vi "VMI_Main_Events.vi"() -> ()   [LabVIEW 2018]
uses:
  <vilib>/vision/Image Controls.llb/IMAQ Image.ctl
  Type defs/TRPES_save_cluster.ctl
  <vilib>/userdefined/High Color/IMAQdx.ctl
  Type defs/Ref_cluster.ctl
  Type defs/Image_info.ctl
  Type defs/PI_delay_settings_alt.ctl
  Type defs/FileAcq_v1_Ctrl.ctl
  Type defs/Scan_ctrl.ctl
  Type defs/VMI_camera_contrl.ctl
  Type defs/DAQ_set_Ctrl.ctl
  Type defs/DAQ_Shutter_Ctrl.ctl
  Type defs/DAQ_AI_Ctrl.ctl
  Type defs/VMI_peak_out.ctl
  Type defs/IO_settings_ctrl.ctl
  Type defs/Header_infor_IF32.ctl
  <vilib>/DAQmx/write.llb/DAQmx Write (Digital 1D Bool NChan 1Samp 1Line).vi
  <vilib>/DAQmx/miscellaneous.llb/DAQmx Fill In Error Info.vi
panel:
  out "Peaks":T1[](array[typedef])
  out "Stage Position":dbl=50.0
  out "Delay Moving":bool
  in  "Files to Save":bool[](array[boolean])
  in  "Shutter2":bool
  in  "Shutter1":bool
  in  "Stop All":bool
  in  "Savechoose":bool caption="Choose save name?"
  out "Autosave?":bool
  in  "Save All":bool
  out "Running":bool
  out "Setup?":bool
  in  "Stop Collect":bool
  in  "New Collect":bool
  in  "Butt_Set":bool
  out "Information":string
  out "Hist_full":dbl[][][](array[numeric])
  in  "Collect":bool
  out "Peak Array":cluster{"X":sgl, "Y":sgl}[][](array[cluster])
  out "size(s) 3":i32
  out "size(s) 2":i32
  out "size(s)":i32
  out "Background 2":cluster{"X":sgl, "Y":sgl}[](array[cluster])
  out "Signal Background":cluster{"X":sgl, "Y":sgl}[](array[cluster])
  out "Background 1":cluster{"X":sgl, "Y":sgl}[](array[cluster])
  out "AI err":dbl[][](array[numeric])
  out "AI in":dbl[][](array[numeric])
  out "Big_image Array":i16[][][](array[numeric])
  out "Histogram_array":i32[][](array[numeric])
  in  "Bakc Image2":i16[][](array[numeric])
  in  "Bakc Image":i16[][](array[numeric])
  in  "Signal Image":i16[][](array[numeric])
  in  "Ref Cluster 1":T2
  out "Session Out":T3
  out "Queue Check":bool
  out "Queue Array":T4[](array[typedef])
  out "Image types Bool":bool[](array[boolean])
  out "Image Set":T5
  out "Points per image":i32[](array[numeric])
  in  "Error In":errorcluster
  out "Error Out":errorcluster
  in  "Tab Control":T6(tab)
  out "Count Rate / s":dbl
  in  "Delay Display":u16(ring) items=["Signal", "Background 1", "Background 2"]
  out "Delay":u8(slide) scale=0.0..4.0
  out "Current Image 3":T5(plugin-control)
  in  "Centroiding":u16(ring) items=["None", "x2"]
  in  "Image Options":u16(ring) items=["Last image", "Real Time", "Summed Image", "Background", "Background 2"]
  in  "Camera Rate / Hz":i32=50
  out "Collection Results":T7
  out "Counts per image":cluster{"X":dbl[], "Y":dbl[]}[](graph)
  in  "Acquire Time":i32=1 caption="How long to Acquire Image / s"
  in  "Total Acquires":i32=10000 caption="How many complete Acquires"
  out "max value":i16
  out "Delay Loop":i32
  out "Total Loop":i32
  in  "Save_Files":cluster{"Files to Save":bool[]}={"Files to Save"=[TRUE, TRUE, TRUE, TRUE]}
  in  "Image Info Acqu":T8={"X size"=782.0, "Y size"=582.0, "Centroiding"=1.0}
  in  "Database":bool
  in  "Log File":bool=TRUE
  in  "Slack":bool
  in  "Delay List":string[][](table)
  out "Delay Scan Steps":i32
  in  "Scan Set up":T9={"Scan Type"=0, "Collection Information File Path"=path "", "Chemical"="Xenon", "Comments"="", "Collection Time / s"=60, "Number Acquires"=1, "How long to acquire"=100} {"Scan Type" items=["Normal Collection - 1 Colour", "Normal Collection - 2 Colour", "Delay Scan - 2 colour", "Accurate Delay Scan - 2 Colour", "Settings file"]}
  in  "Collection Information":T10[](array[typedef])=[{"Type"="Signal and Background", "LaserWave1"=0.0, "Shutter1"=TRUE, "LaserWave2"=0.0, "Shutter2"=FALSE, "FileEnd"="_SignalBack", "Collect"=TRUE}]
  in  "Delay Cluster":T11={"System no."=0, "Identification"="", "Device ID out"=0, "Postion / mm"=[], "SN out"="", "Movement Range"=[], "Conn. Axes"=[], "Target Position / mm"=50.0, "Velocity / mm s^-1"=0.15, "Set-up"=FALSE, "Moving"=FALSE, "Step Size / mm "=0.15, "Stage Number"=0, "Polling Time /ms"=0, "Delay Scan?"=FALSE, "Accurate Scan"=FALSE, "CmdMovDelay"=FALSE, "CmdStopDelay"=FALSE, "Delay List"=[["Number", "Target / mm", "Relative Integration Time"]], "Scan Start /mm"=50.0, "Scan End / mm"=80.0}
  in  "Save Options":T12={"Auto Save"=FALSE, "Main Directory"=path "C:/Data", "Current File Date and endings"="", "Save Path"=path "C:/Data", "Backup Path"=path "Z:/Research_Projects/Photochemistry", "Extra Dir Information"="", "Remote"=TRUE}
  out "Last Slack":string
  in  "Loops per Save":i32
  in  "DAQ Settings":T13={"Shutters Settings"=[{"Name"="Shutter 1", "DAQ Channel/line"="Dev1/port0/line0", "Active"=TRUE}, {"Name"="Shutter 2", "DAQ Channel/line"="Dev1/port0/line1", "Active"=TRUE}], "Shutter Task"="Shutters_spare", "Acquire Settings"=[{"Name"="Power", "DAQ Channel/line"="Dev1/ai0", "Max V"=5.0, "Min V"=-5.0, "input terminal configuration"=10106, "Active"=TRUE}, {"Name"="Pressure 1", "DAQ Channel/line"="Dev1/ai1", "Max V"=5.0, "Min V"=-5.0, "input terminal configuration"=10106, "Active"=TRUE}, {"Name"="Pressure 2", "DAQ Channel/line"="Dev1/ai2", "Max V"=5.0, "Min V"=-5.0, "input terminal configuration"=10106, "Active"=TRUE}], "AI Task"="Acquire", "Sample mode"=10123, "Number of Samples"=100, "Rate"=1000.0, "AI Name"="Acquire", "DO Name"="Shutters"} {"Sample mode" items=["Finite Samples"=10178, "Continuous Samples"=10123, "Hardware Timed Single Point"=12522]; "Acquire Settings"."input terminal configuration" items=["default"=-1, "RSE"=10083, "NRSE"=10078, "Differential"=10106, "Pseudodifferential"=12529]}
  in  "Camera Settings":T16={"Run Options"=0, "Run Mode"=0, "Attributes"="[NIIMAQ_HEADER]\nType = 2\nVersion = 8\n\n[CAMERA_DATA]\nAcquisitionAttributes::VideoMode = \"Format 7, Mode 0, 782 x 582\"\nAcquisitionAttributes::OffsetX = \"0\"\nAcquisitionAttributes::OffsetY = \"0\"\nAcquisitionAttributes::Width = \"782\"\nAcquisitionAttributes::Height = \"582\"\nAcquisitionAttributes::Bayer::Algorithm = \"Bilinear\"\nAcquisitionAttributes::Bayer::GainB = \"1\"\nAcquisitionAttributes::Bayer::GainG = \"1\"\nAcquisitionAttributes::Bayer::GainR = \"1\"\nAcquisitionAttributes::Bayer::Pattern = \"Use hardware value\"\nAcquisitionAttributes::BitsPerPixel = \"Use hardware value\"\nAcquisitionAttributes::Controller::DesiredStreamChannel = \"0\"\nAcquisitionAttributes::Controller::StreamChannelMode = \"Automatic\"\nAcquisitionAttributes::IgnoreFirstFrame = \"false\"\nAcquisitionAttributes::ImageDecoderCopyMode = \"Auto\"\nAcquisitionAttributes::OutputImageType = \"Auto\"\nAcquisitionAttributes::OverwriteMode = \"Get Newest\"\nAcquisitionAttributes::PixelSignedness = \"Signed\"\nAcquisitionAttributes::ReceiveTimestampMode = \"None\"\nAcquisitionAttributes::ReserveDualPackets = \"false\"\nAcquisitionAttributes::ShiftPixelBits = \"false\"\nAcquisitionAttributes::Speed = \"400 Mbps\"\nAcquisitionAttributes::SwapPixelBytes = \"false\"\nAcquisitionAttributes::Timeout = \"5000\"\nCameraAttributes::Brightness::Mode = \"Relative\"\nCameraAttributes::Gain::Mode = \"Relative\"\nCameraAttributes::Shutter::Mode = \"Relative\"\nCameraAttributes::Brightness::Value = \"16\"\nCameraAttributes::Gain::Value = \"600\"\nCameraAttributes::Shutter::Value = \"700\"\nCameraAttributes::Trigger::TriggerMode = \"Off\"\nCameraAttributes::Trigger::TriggerActivation = \"Level High\"\nCameraAttributes::Trigger::TriggerSource = \"Source 0\"\n", "Peak Find Settings"={"Objects"=0, "Threshold"=10, "Reject Border"=FALSE, "Fill Holes"=FALSE, "Min Object Size"=FALSE, "Min Size"=3, "Max Object Size"=FALSE, "Max Size"=100, "Show Search Area"=FALSE, "Show Center"=FALSE, "Show Bounding Box"=FALSE}, "Image Type"=0, "Test Image File Path"=path "C:/Users/Parkes/Documents/GitHub/Camera-Acquire_Labview/mcp_hit_test.png", "Camera Name"="cam0", "X Size"=782.0, "Y Size"=582.0} {"Image Type" items=["Grayscale (U8)", "Grayscale (I16)", "Grayscale (SGL)", "Complex (CSG)", "RGB (U32)", "HSL (U32)", "RGB (U64)", "Grayscale (U16)"]; "Peak Find Settings"."Objects" items=["Bright Objects", "Dark Objects"]; "Peak Find Settings"."Threshold" min=1 max=999999999 step=1; "Peak Find Settings"."Max Size" min=1 max=999999999 step=1; "Peak Find Settings"."Min Size" min=1 max=999999999 step=1; "Run Mode" items=["Simple Collect", "Collect Images", "Delay Scan"]; "Run Options" items=["Collect Camera", "Test with Image"]}
  in  "Analysis Path":path
  in  "Save anl":bool
  in  "Stop All Anly":bool
  out "Loaded":bool
  in  "Butt_Load":bool
  out "Num Points":i32
  out "Loaded Points":cluster{"X":sgl, "Y":sgl}[](array[cluster])
  out "Image Array":i16[][](array[numeric])
  in  "Image Info":T8={"X size"=782.0, "Y size"=582.0, "Centroiding"=1.0}
  out "Intensity Graph":dbl[][](graph)
  # "Peak List"
  # "Histogram"
  # "Full Histogram"
  # "Images"
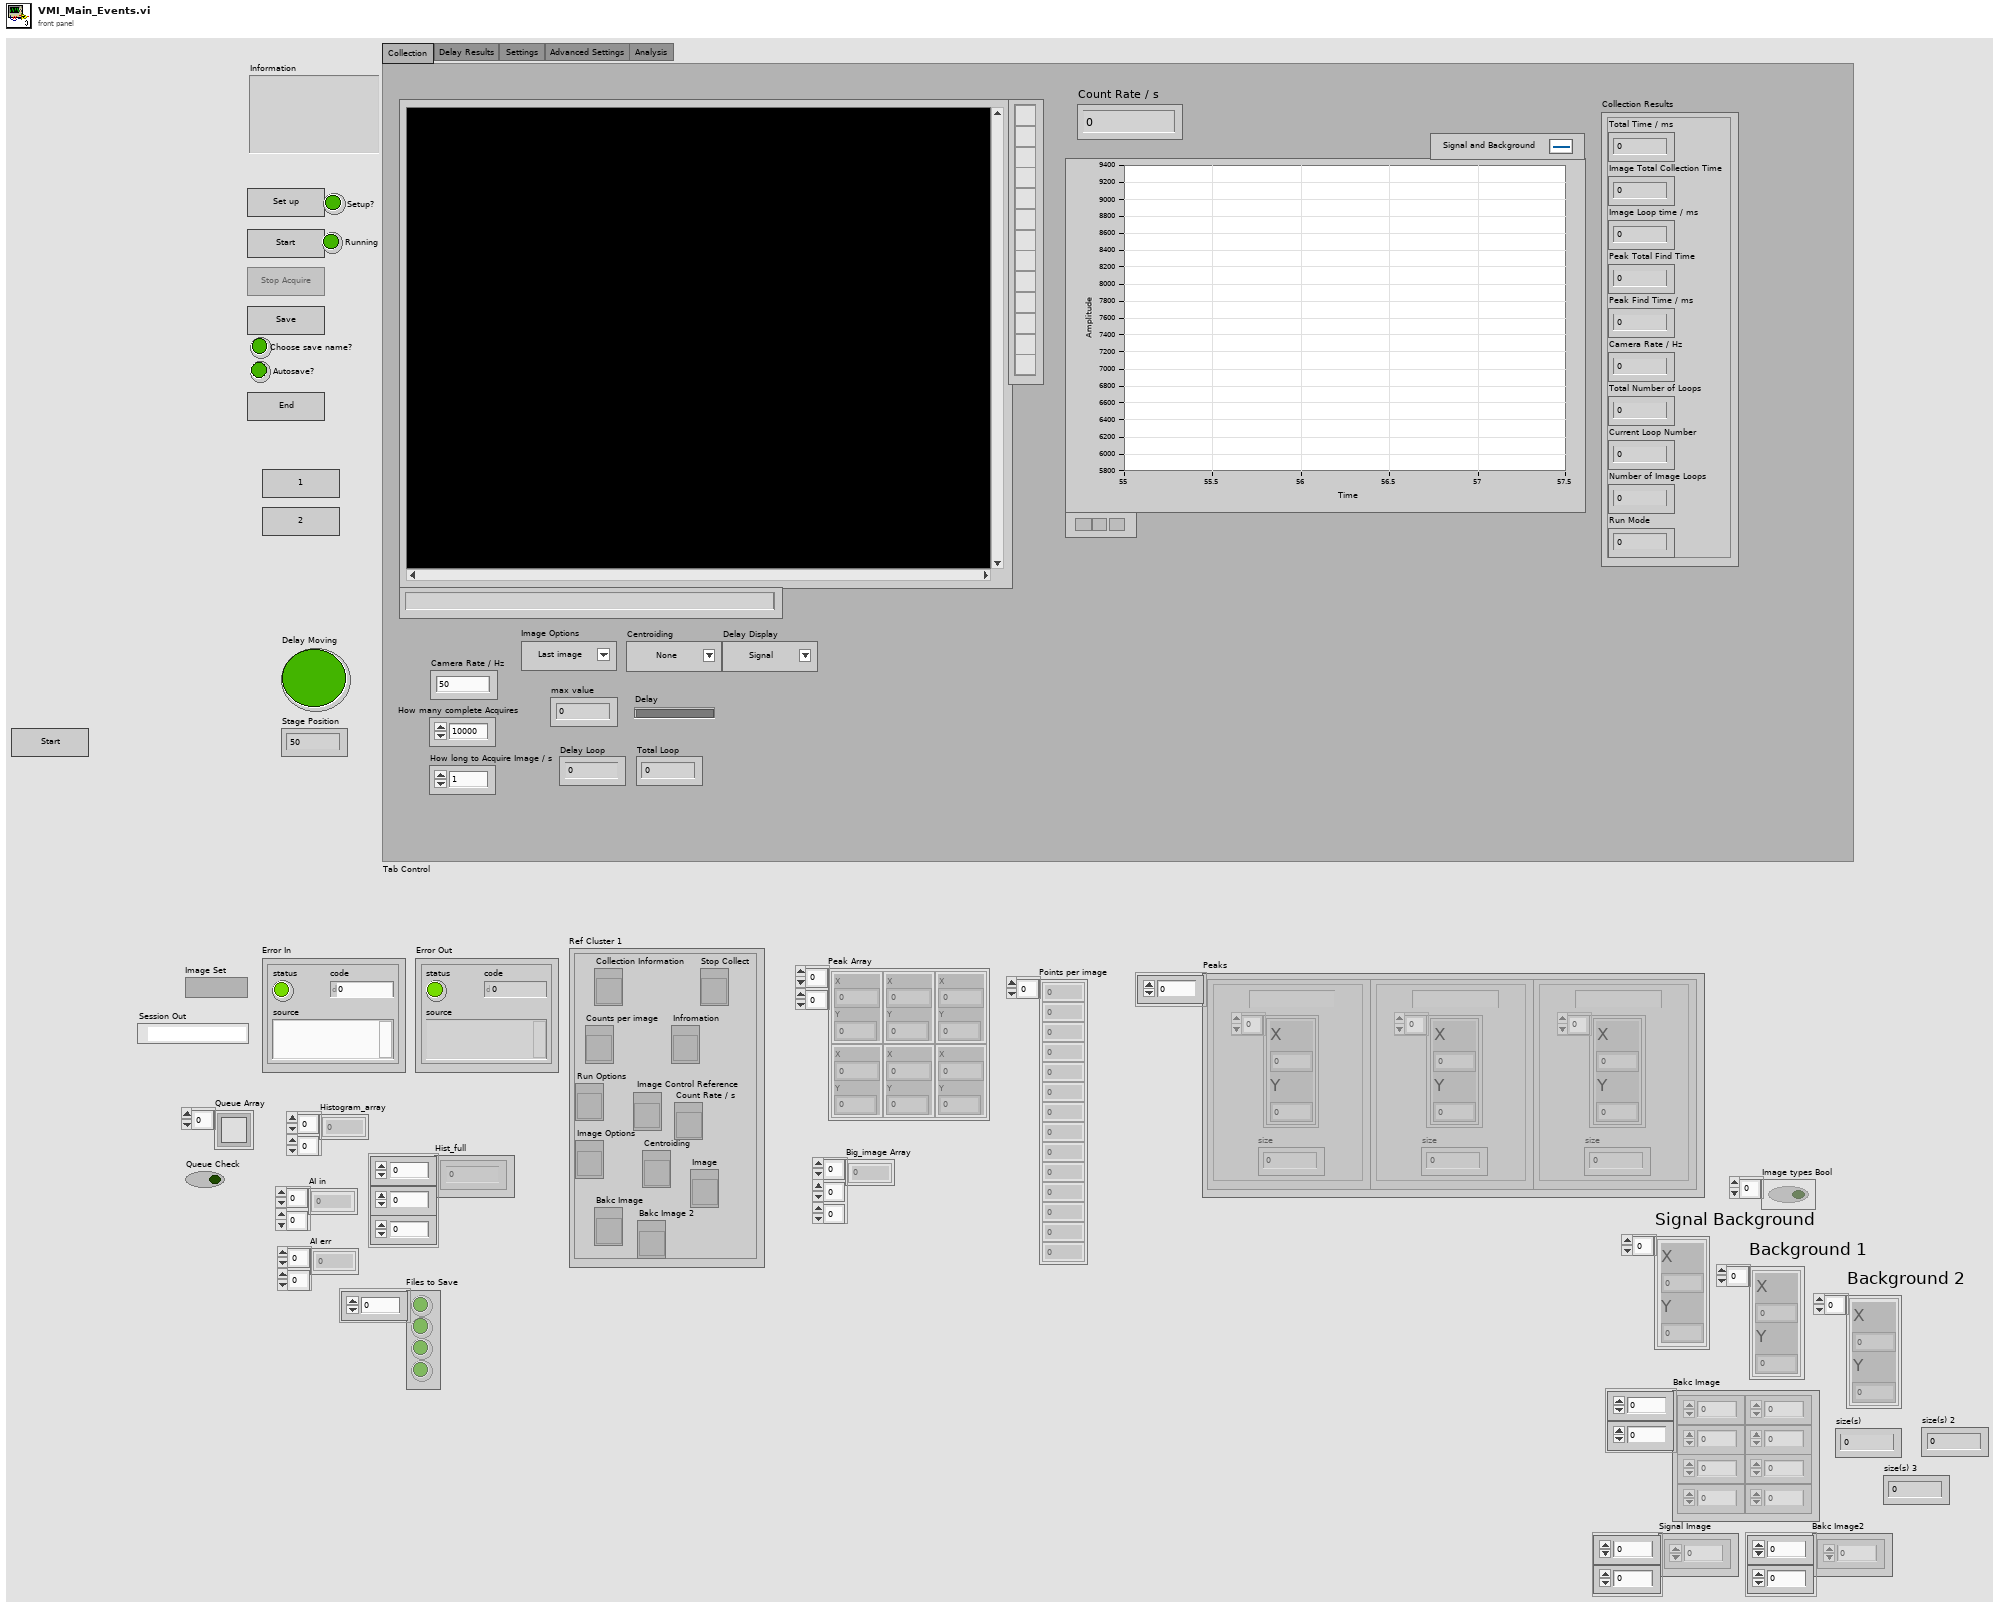
[diagram p1: front panel]
types:
  T1 = typedef "VMI_peak_out.ctl" = cluster{"Peaks":cluster{"X":sgl, "Y":sgl}[], "size":i32, "Title":string}
  T2 = typedef "Ref_cluster.ctl" = cluster{"Stop Collect ":refnum<vi>, "Collection Information ":refnum<vi>, "Infromation":refnum<vi>, "Counts per image":refnum<vi>, " Image Control Reference ":refnum<vi>, "Run Options":refnum<vi>, "Image Options":refnum<vi>, "Centroiding":refnum<vi>, "Image":refnum<vi>, "Bakc Image":refnum<vi>, "Bakc Image 2":refnum<vi>, "Count Rate / s":refnum<vi>}
  T3 = typedef "IMAQdx.ctl" = refnum<k21>
  T4 = typedef "Queue RefNum" = refnum<k1>
  T5 = typedef "IMAQ Image.ctl" = refnum<image>
  T6 = enum32{"Collection", "Delay Results", "Settings ", "Advanced Settings", "Analysis"}
  T7 = cluster{"Total Time / ms":dbl, "Image Total Collection Time":dbl, "Image Loop time / ms":dbl, "Peak Total Find Time":dbl, "Peak Find Time / ms":dbl, "Camera Rate / Hz":dbl, "Total Number of Loops":dbl, "Current Loop Number":dbl, "Number of Image Loops":dbl, "Run Mode":dbl}
  T8 = typedef "Image_info.ctl" = cluster{"X size":dbl, "Y size":dbl, "Centroiding":dbl}
  T9 = typedef "Scan_ctrl.ctl" = cluster{"Scan Type":u16, "Collection Information File Path":path, "Chemical":string, "Comments":string, "Collection Time / s":i32, "Number Acquires":i32, "How long to acquire":i32}
  T10 = typedef "FileAcq_v1_Ctrl.ctl" = cluster{"Type":string, "LaserWave1":dbl, "Shutter1":bool, "LaserWave2":dbl, "Shutter2":bool, "FileEnd":string, "Collect":bool}
  T11 = typedef "PI_delay_settings_alt.ctl" = cluster{"System no.":i32, "Identification":string, "Device ID out":i32, "Postion / mm":dbl[], "SN out":string, "Movement Range":dbl[], "Conn. Axes":string[], "Target Position / mm":dbl, "Velocity / mm s^-1":dbl, "Set-up":bool, "Moving":bool, "Step Size / mm ":dbl, "Stage Number":i32, "Polling Time /ms":i32, "Delay Scan?":bool, "Accurate Scan":bool, "CmdMovDelay":bool, "CmdStopDelay":bool, "Delay List":string[][], "Scan Start /mm":dbl, "Scan End / mm":dbl}
  T12 = typedef "TRPES_save_cluster.ctl" = cluster{"Auto Save":bool, "Main Directory":path, "Current File Date and endings":string, "Save Path":path, "Backup Path":path, "Extra Dir Information":string, "Remote":bool}
  T13 = typedef "DAQ_set_Ctrl.ctl" = cluster{"Shutters Settings":T14[], "Shutter Task":refnum<k21>, "Acquire Settings":T15[], "AI Task":refnum<k21>, "Sample mode":i32, "Number of Samples":i32, "Rate":dbl, "AI Name":string, "DO Name":string}
  T14 = typedef "DAQ_Shutter_Ctrl.ctl" = cluster{"Name":string, "DAQ Channel/line":string, "Active":bool}
  T15 = typedef "DAQ_AI_Ctrl.ctl" = cluster{"Name":string, "DAQ Channel/line":string, "Max V":dbl, "Min V":dbl, "input terminal configuration":i32, "Active":bool}
  T16 = typedef "VMI_camera_contrl.ctl" = cluster{"Run Options":u16, "Run Mode":u16, "Attributes":string, "Peak Find Settings":cluster{"Objects":u16, "Threshold":i32, "Reject Border":bool, "Fill Holes":bool, "Min Object Size":bool, "Min Size":i32, "Max Object Size":bool, "Max Size":i32, "Show Search Area":bool, "Show Center":bool, "Show Bounding Box":bool}, "Image Type":T17, "Test Image File Path":path, "Camera Name":string, "X Size":dbl, "Y Size":dbl}
  T17 = typedef "Image Type" = u32
  T18 = enum8{"Enabled", "Disabled", "Disabled and Grayed Out"}
  T19 = typedef "IO_settings_ctrl.ctl" = cluster{"IMAQ In":T5, "Camera Session":T3, "Shutter Task":refnum<k21>, "AI task":refnum<k21>}
  T20 = cluster{"Collection Information":T10[], "ChangeFile":bool, "Image Info":T8, "SAve Paths":path[], "Save":bool[], "Current File Date":string}
  T21 = cluster{"Peak Array All":cluster{"X":sgl, "Y":sgl}[][][], "AI per delay All":dbl[][][], "Counts per delay All":dbl[][][], "Std per delay All":dbl[][][], "Hit x":dbl[][]}
  T22 = typedef "Header_infor_IF32.ctl" = cluster{"File Name":string, "Time":string, "Date":string, "Size":string}
  T23 = cluster{"Objects":u16, "Threshold":i32, "Reject Border":bool, "Fill Holes":bool, "Min Object Size":bool, "Min Size":i32, "Max Object Size":bool, "Max Size":i32, "Show Search Area":bool, "Show Center":bool, "Show Bounding Box":bool}
  T24 = typedef "Database_control.ctl" = cluster{"filename":string, "date":string, "type":string, "chemical":string, "experiment":string, "laser1":dbl, "laser2":dbl}
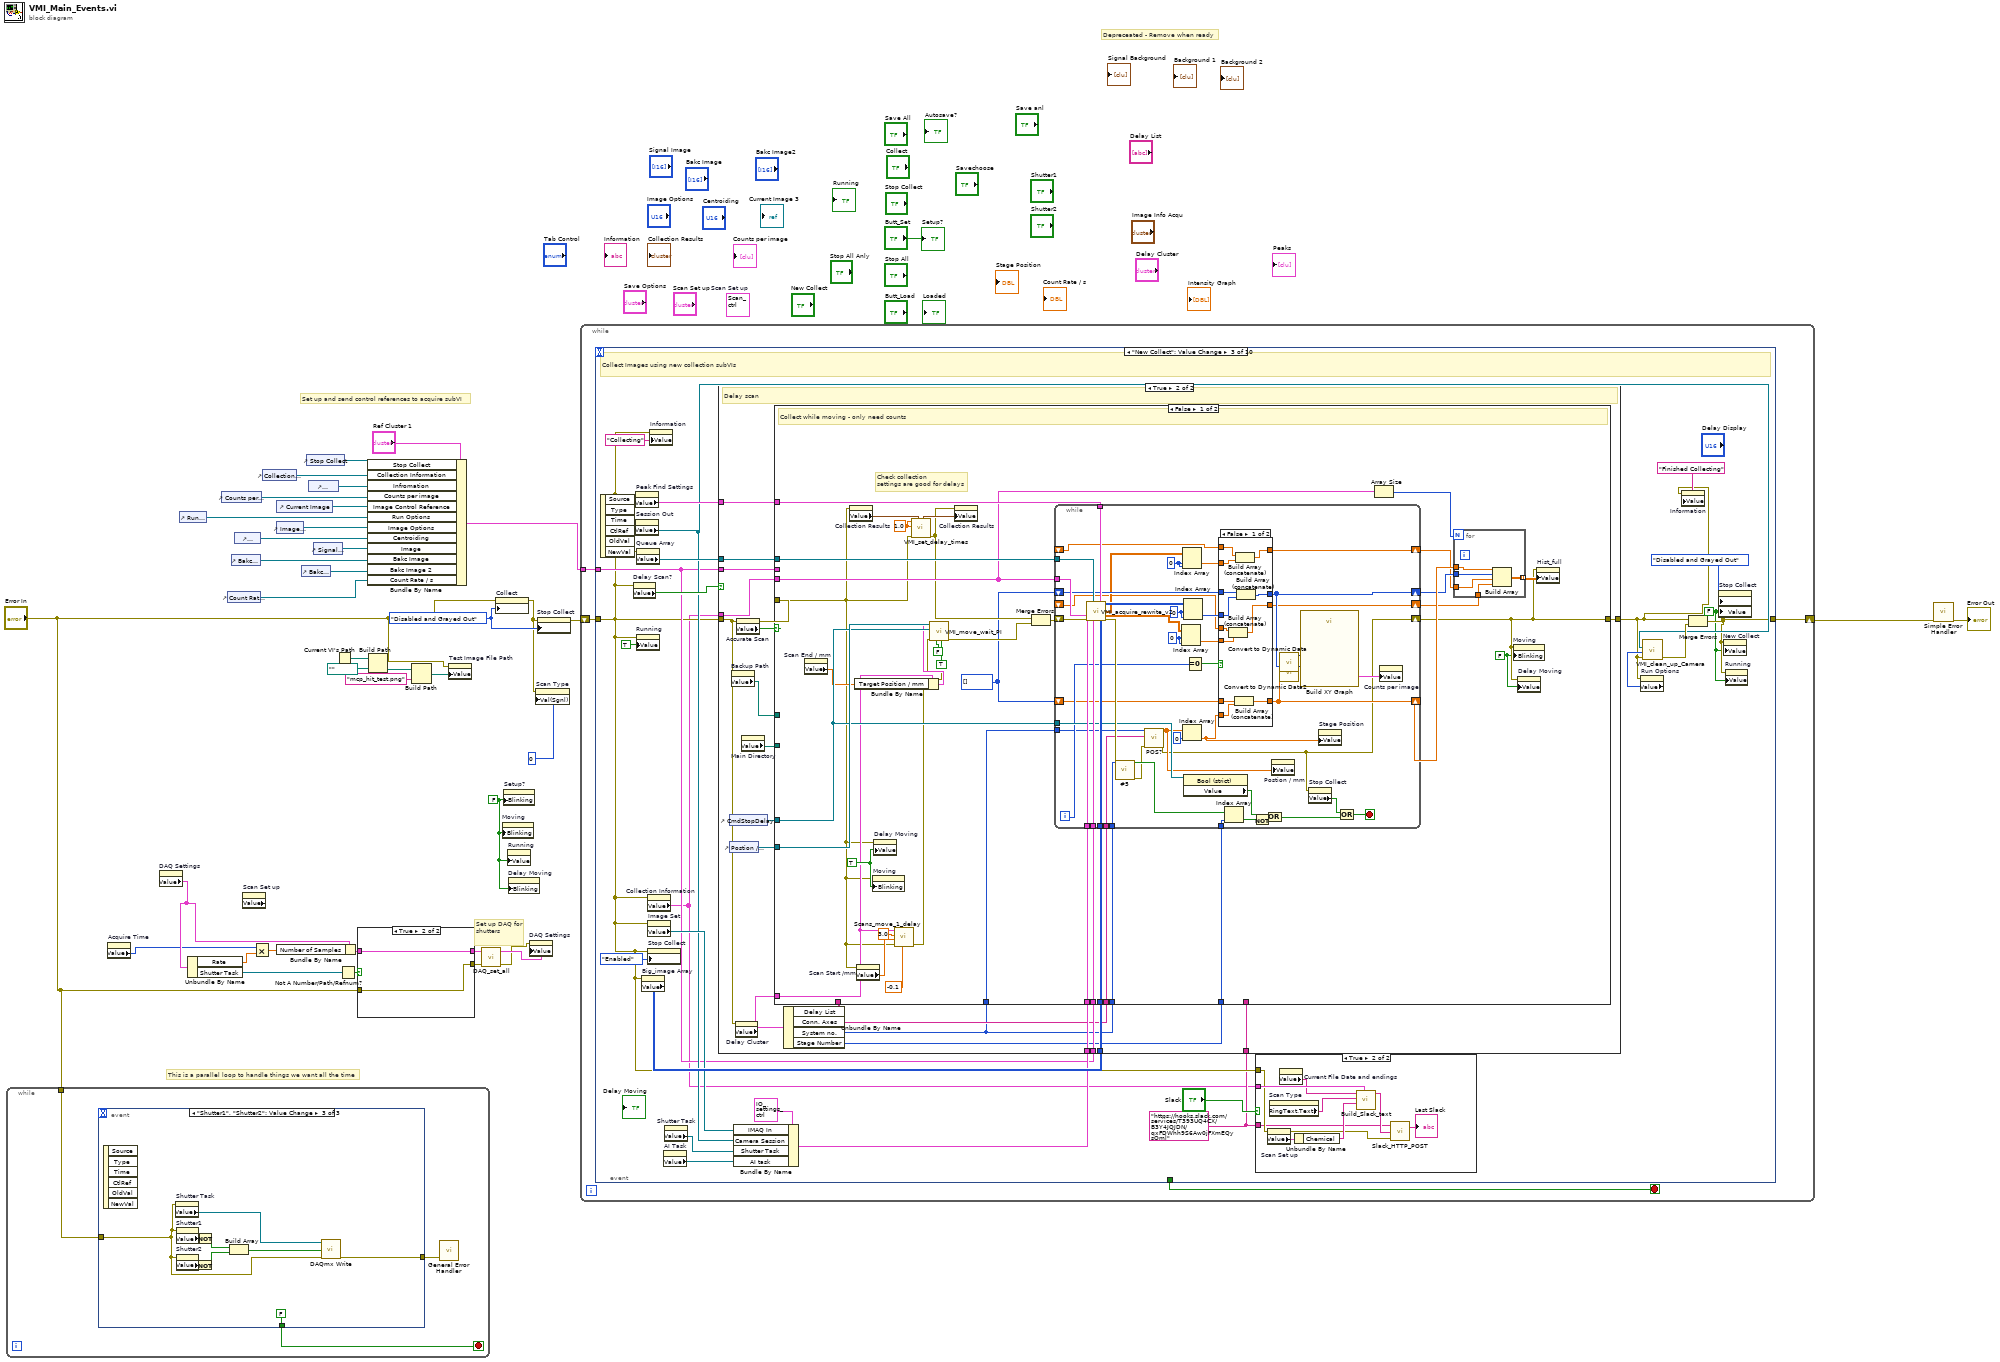
[diagram p0: block diagram]
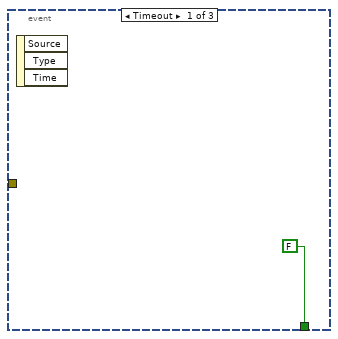
[diagram p2: hidden frame]
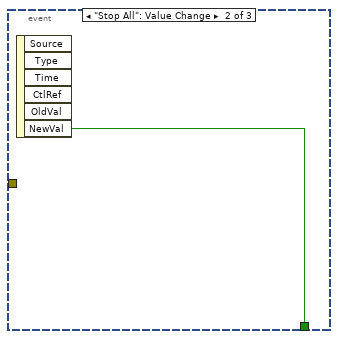
[diagram p3: hidden frame]
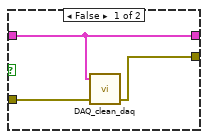
[diagram p4: hidden frame]
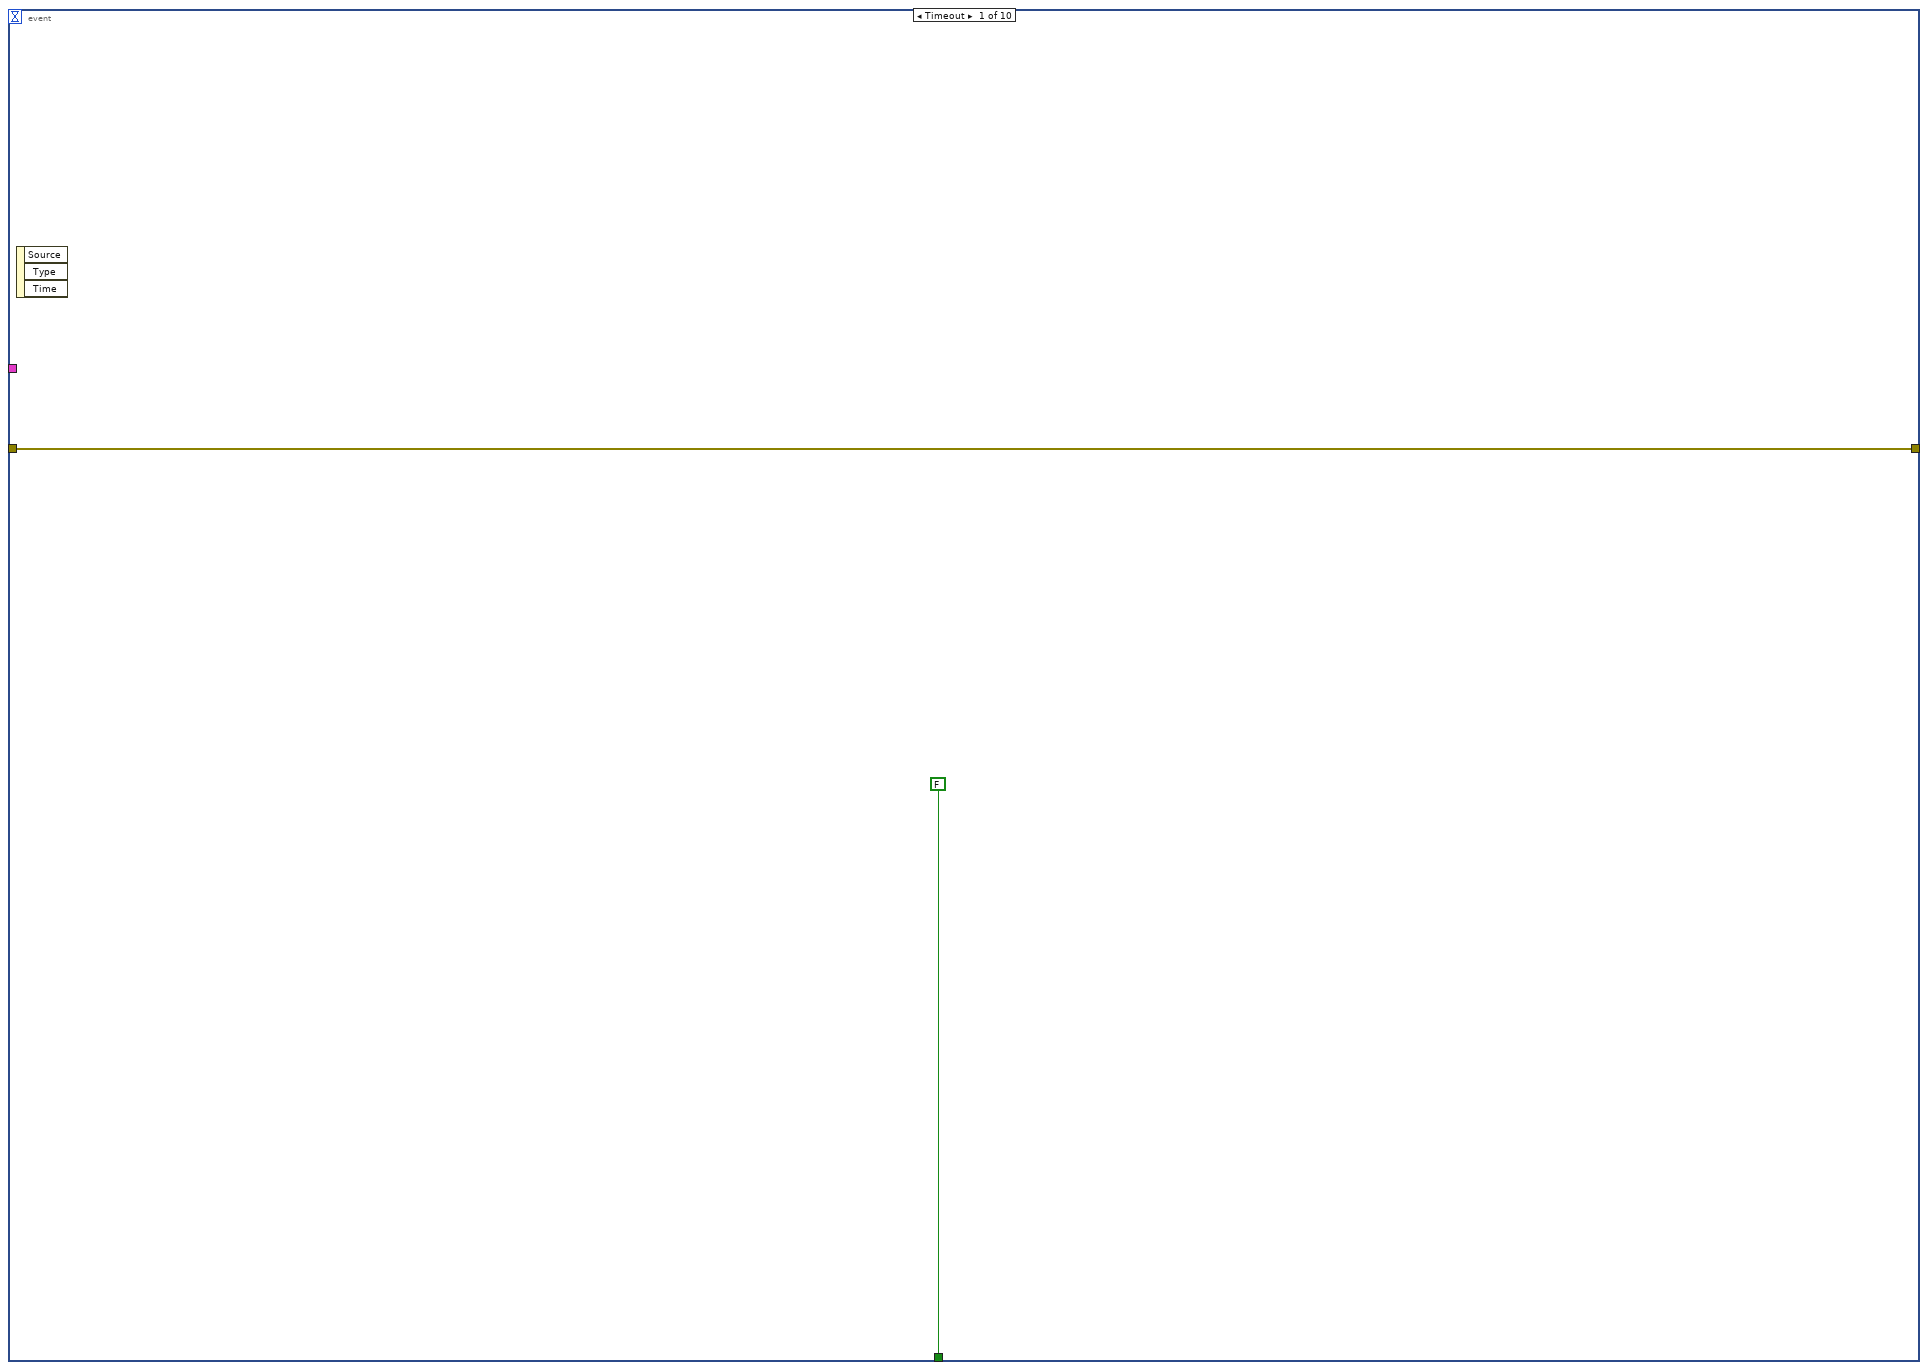
[diagram p5: hidden frame]
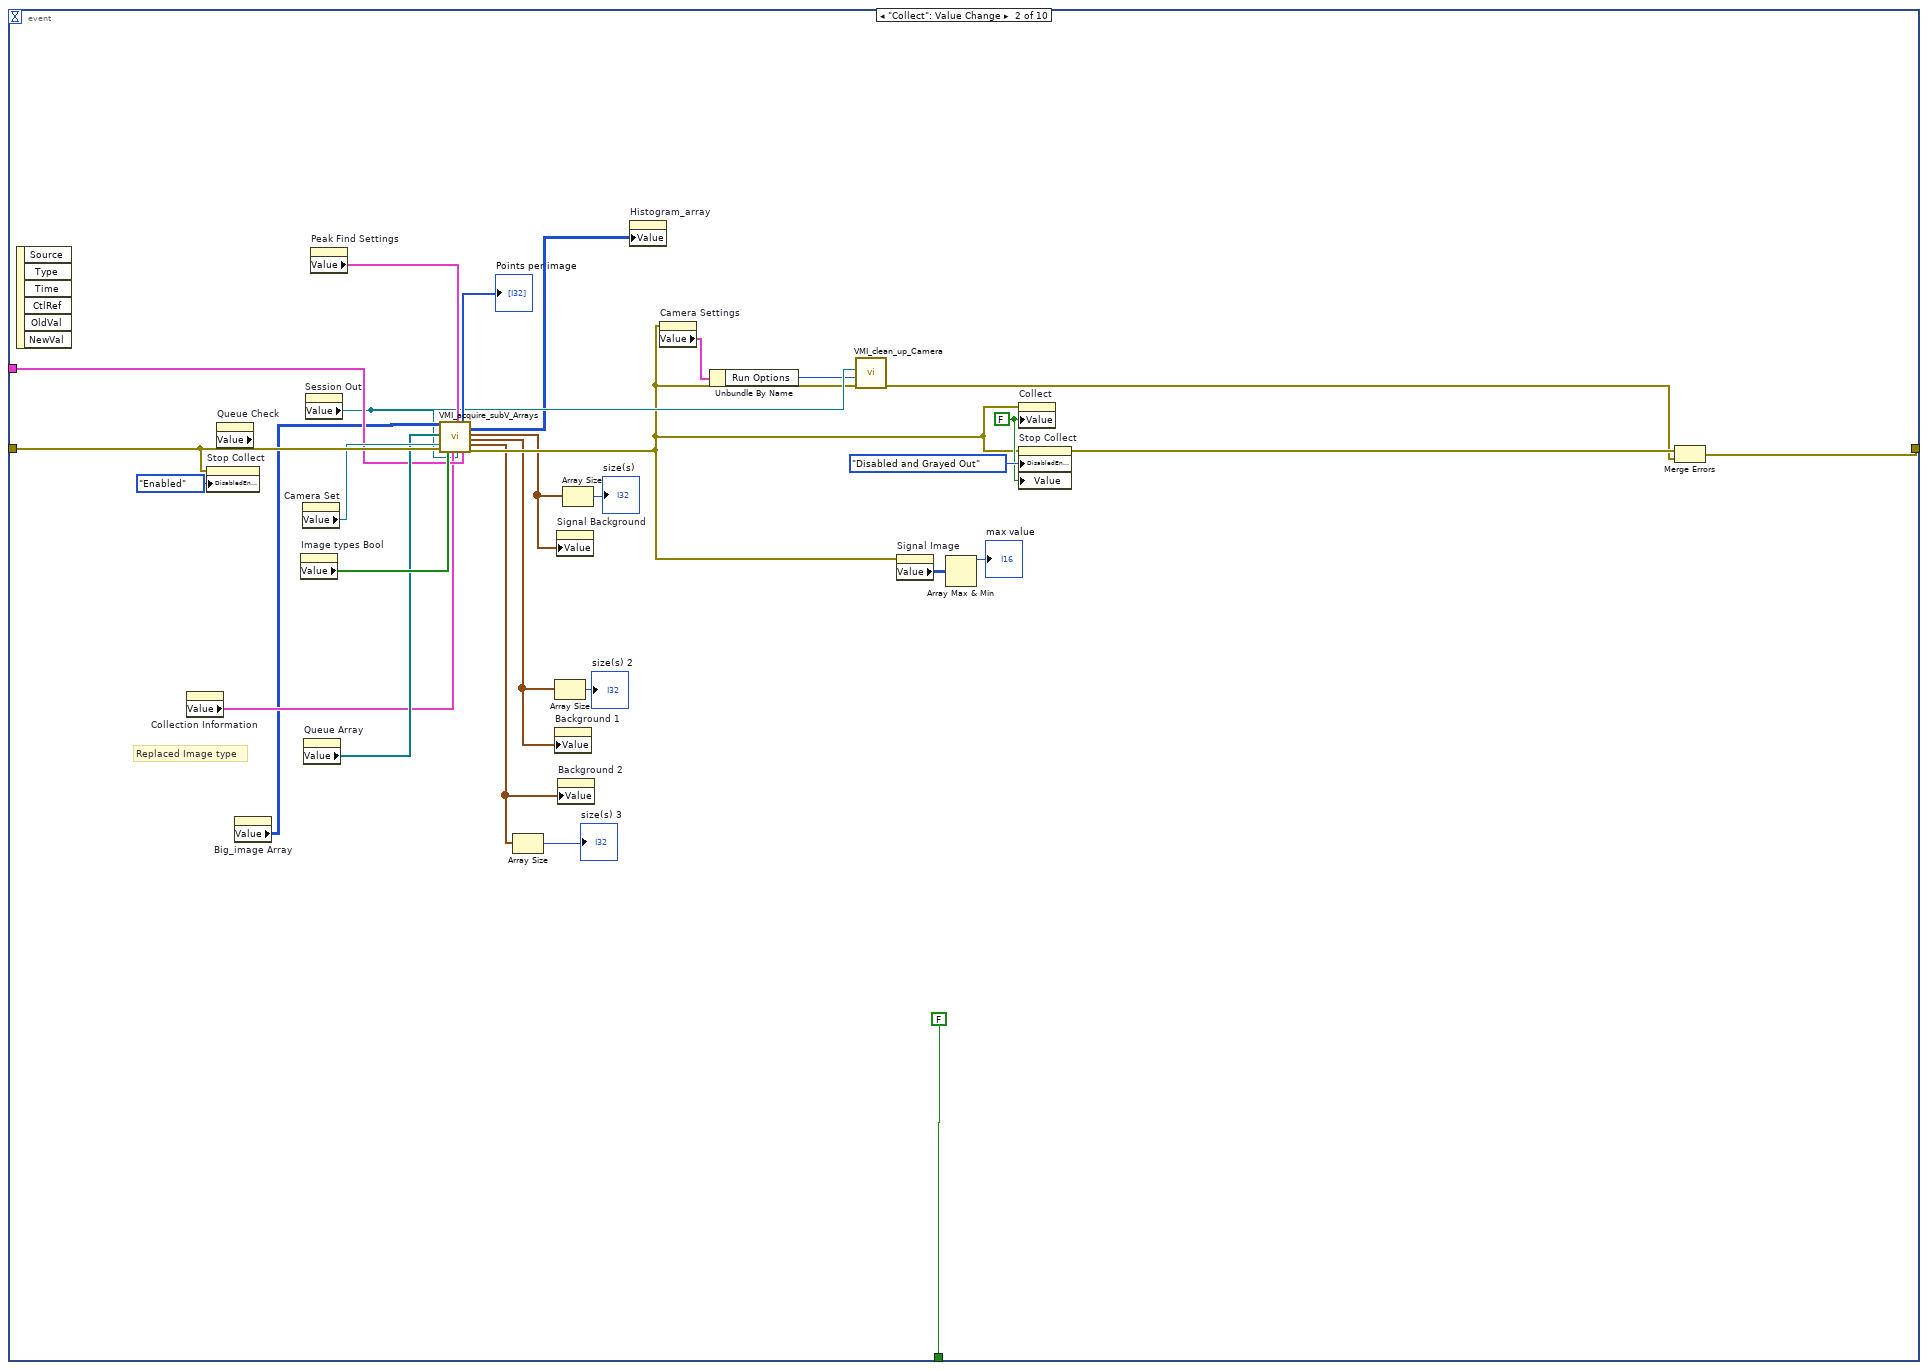
[diagram p6: hidden frame]
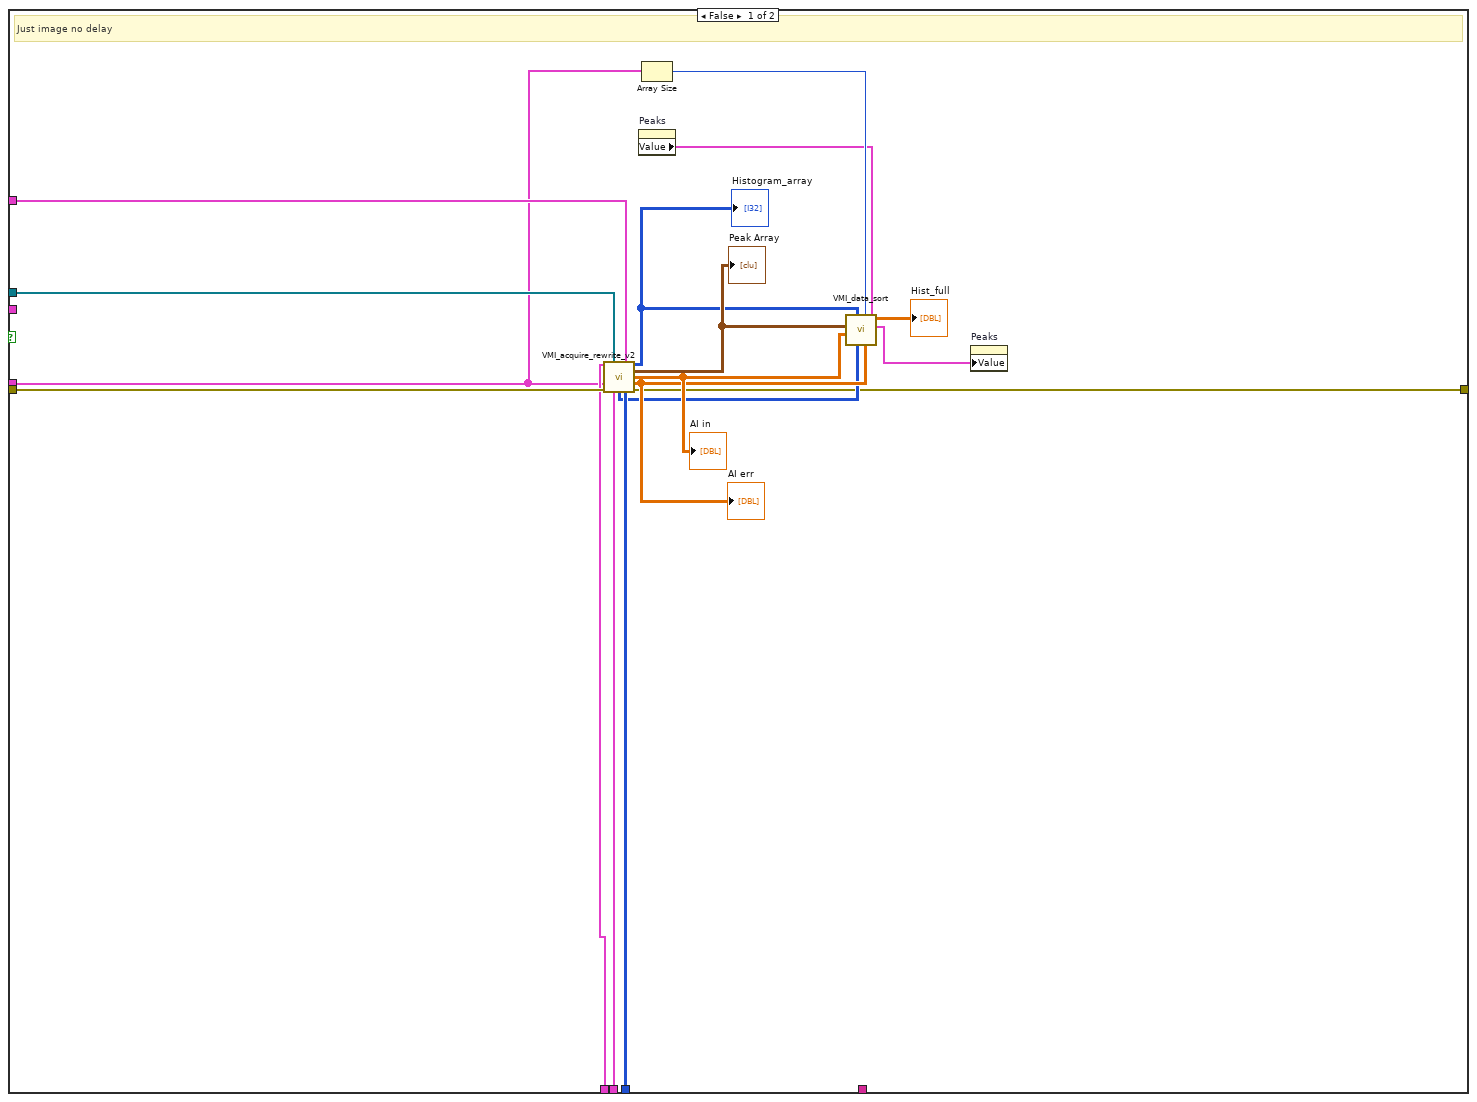
[diagram p8: hidden frame]
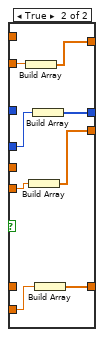
[diagram p9: hidden frame]
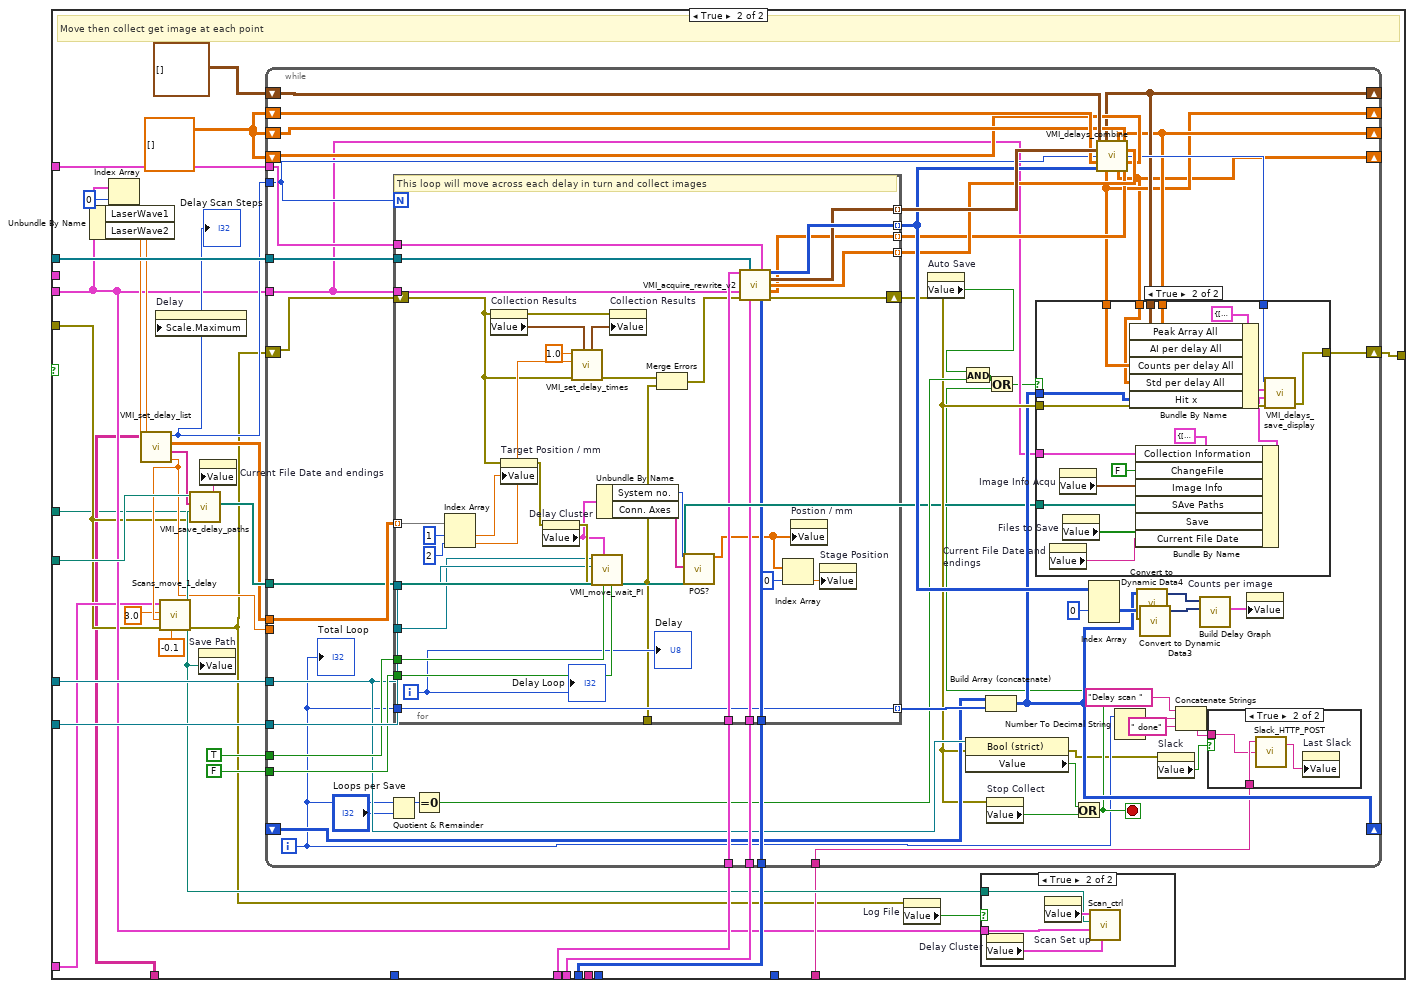
[diagram p10: hidden frame]
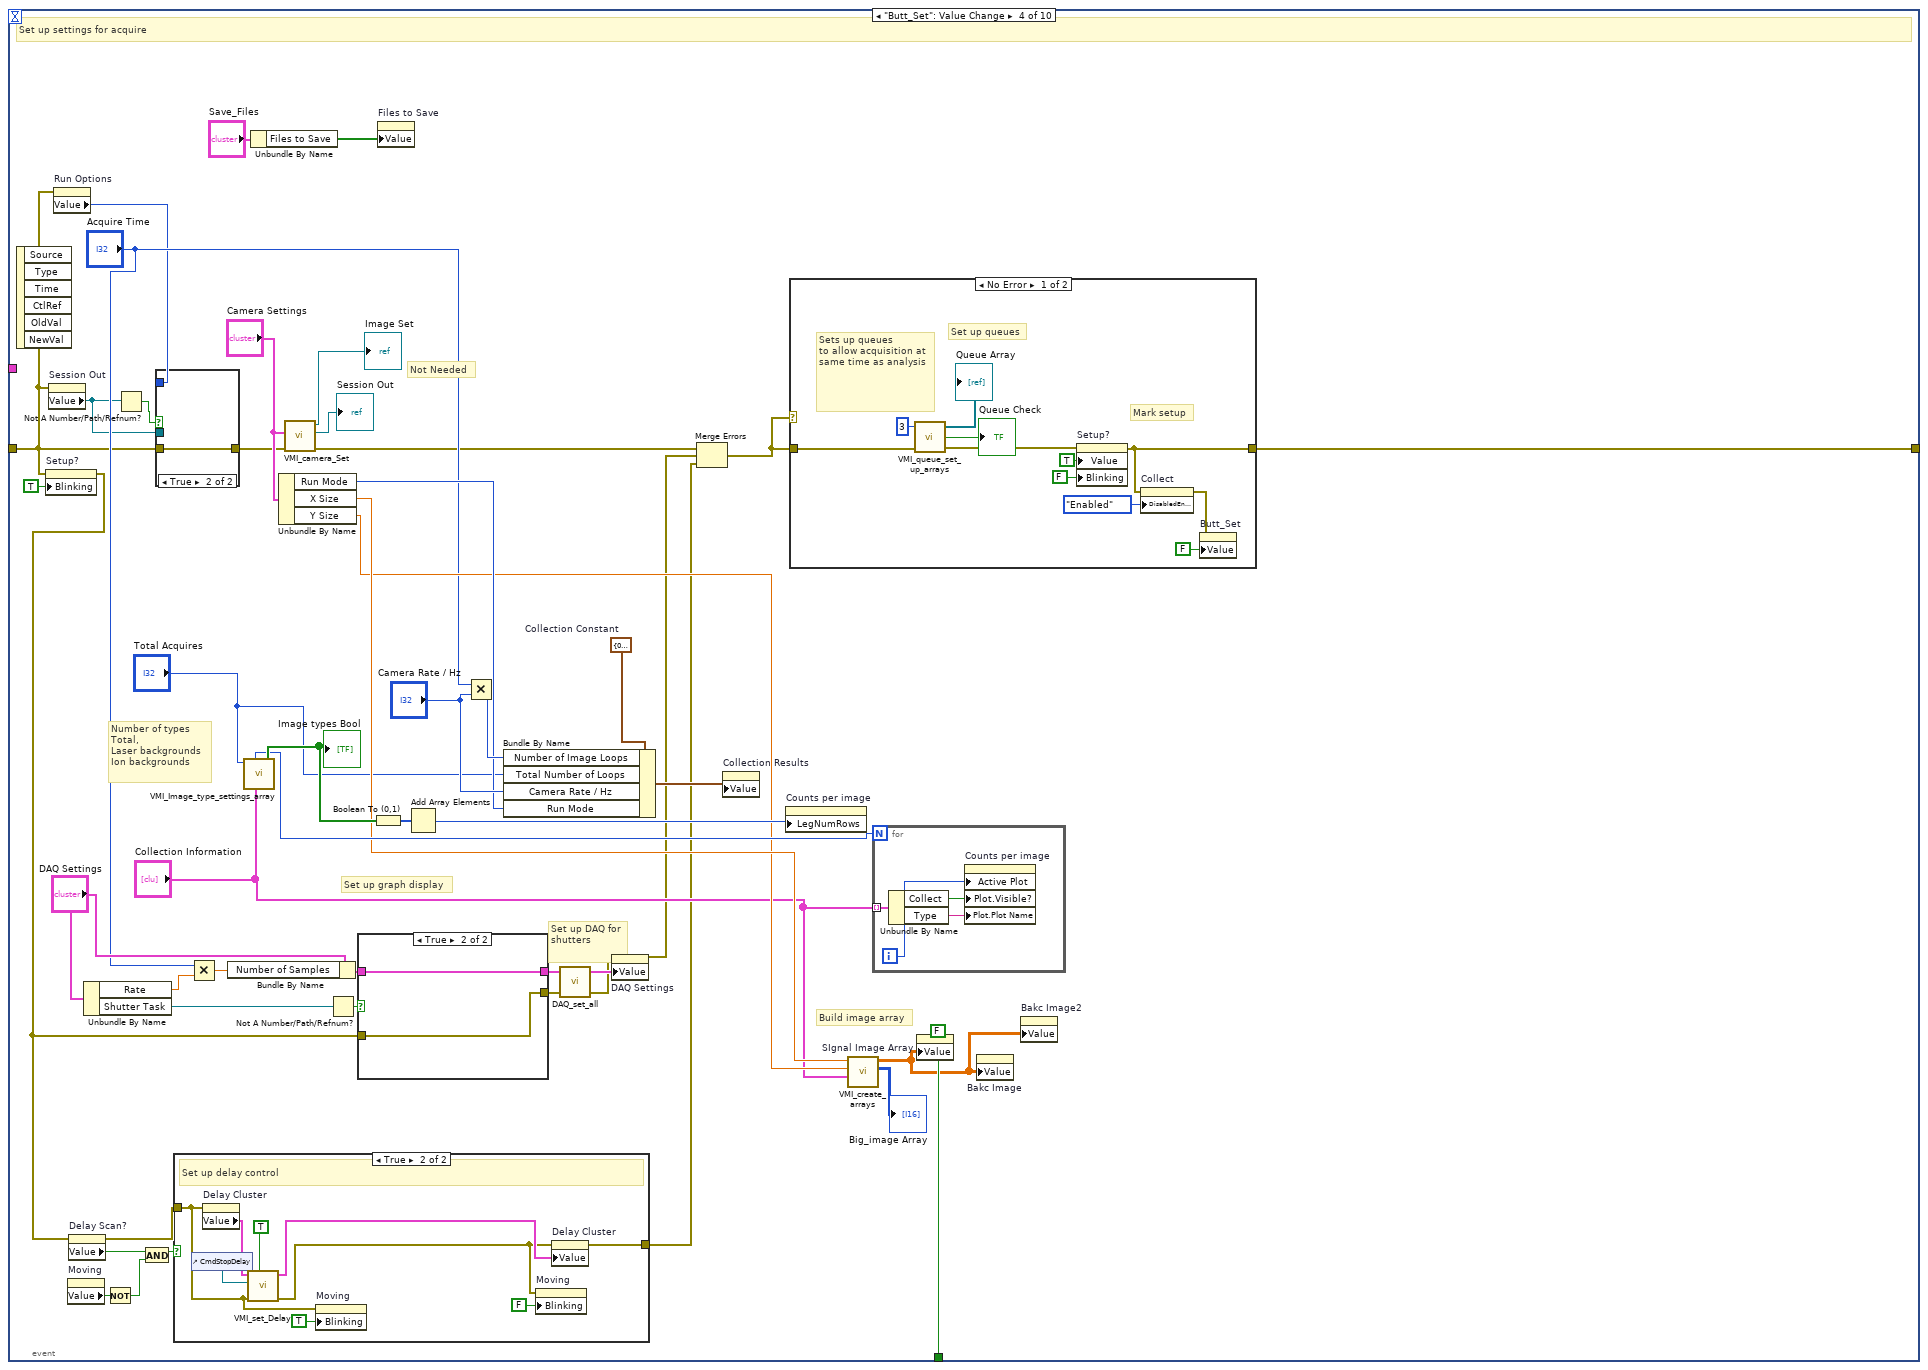
[diagram p14: hidden frame]
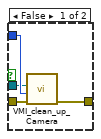
[diagram p15: hidden frame]
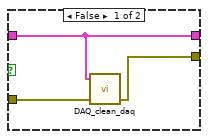
[diagram p16: hidden frame]
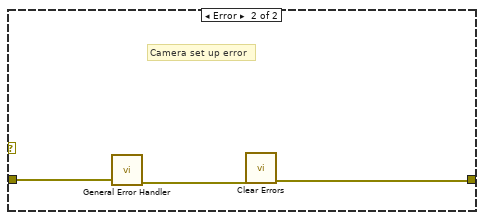
[diagram p18: hidden frame]
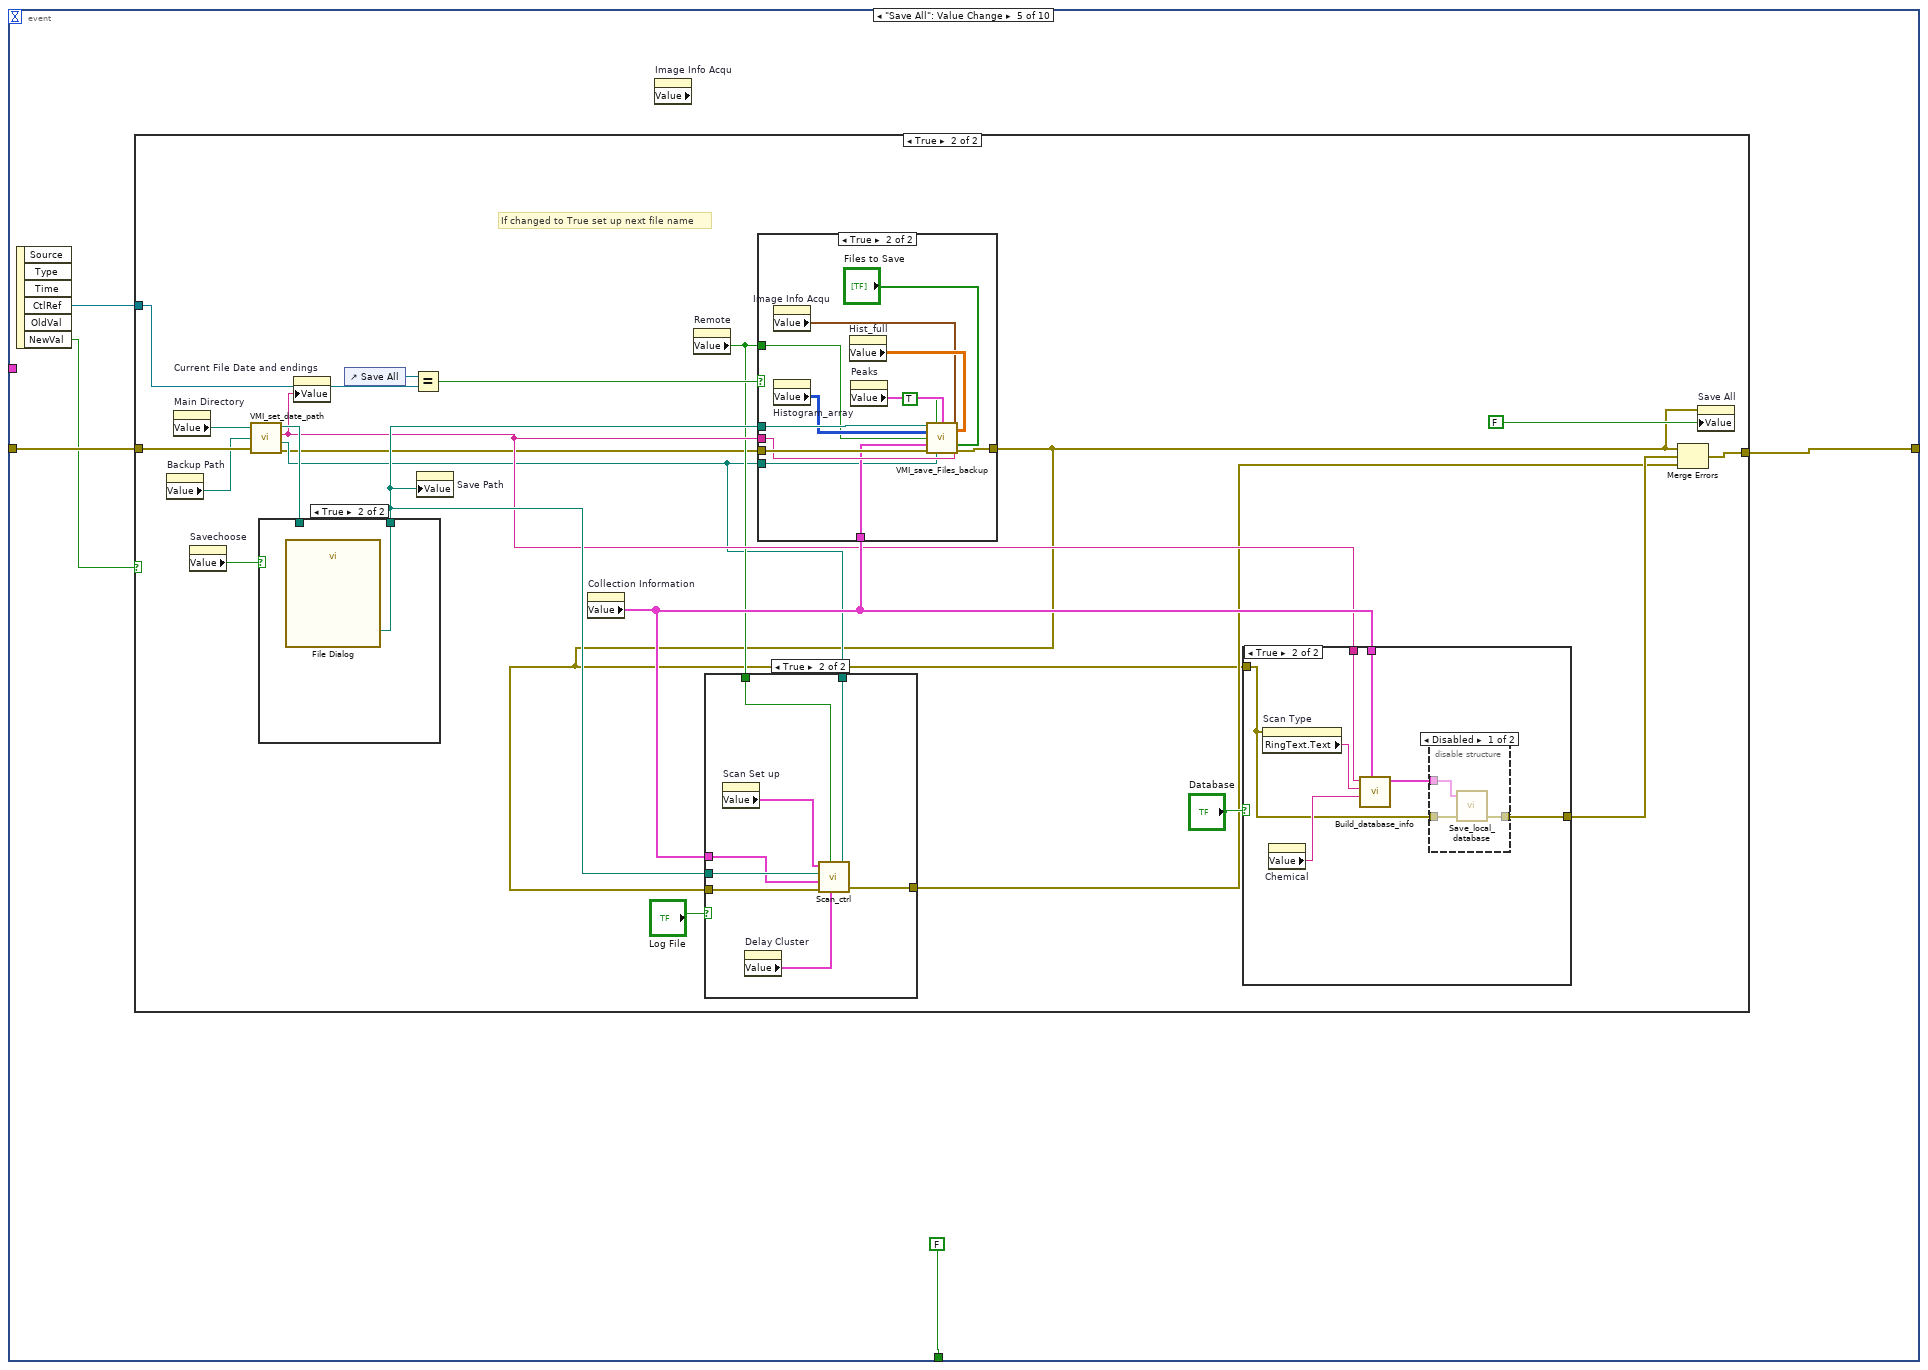
[diagram p19: hidden frame]
diagram:
  w14 = FALSE ("Blinking")
  (unwired) T9 {"Scan Type"=0, "Collection Information File Path"=path "", "Chemical"="Xenon", "Comments"="", "Collection Time / s"=60, "Number Acquires"=1, "How long to acquire"=100}  # Scan Set up
  w37 = T18."Disabled and Grayed Out" ("Disabled")
  # "This is a parallel loop to handle things we want all the time"
  # "Set up DAQ for shutters"
  # "Depreceated - Remove when ready"
  # "Set up and send control references to acquire subVI"
  n1 = while {
    tunnel: "Error In" -> [w41]
    stop <- w42 stop-if-true
    n2 = event shown="[2] \"Shutter1\", \"Shutter2\": Value Change" {
      selector: _ -> [_ _ _]
      dyn-events: _ -> [_ _ _]
      timeout: _ -> [_ _ _]
      tunnel: [FALSE w44 FALSE ("NewVal")] -> w42
      tunnel: w41 -> [_ _ w47]
      tunnel: [_ _ w45] -> w40
      event Timeout {
        n3 = event-data() -> ()  [unwired: 1 in, 3 out]
      }
      event "Stop All": Value Change {
        n4 = event-data() -> ("NewVal"=w44:bool)  [unwired: 1 in, 5 out]
      }
      event "Shutter1", "Shutter2": Value Change {
        n5 = event-data() -> ()  [unwired: 1 in, 6 out]
        n6 = property on="Shutter Task" class="DAQmxName (strict)"(error in=w47) -> ("Value"=w51:refnum<k21>)  [unwired: 1 in, 2 out]
        n7 = property on="Shutter1" class="Bool (strict)"(error in=w47) -> ("Value"=w48:bool)  [unwired: 1 in, 2 out]
        n8 = property on="Shutter2" class="Bool (strict)"(error in=w47) -> ("Value"=w49:bool)  [unwired: 1 in, 2 out]
        n9 = Not(x=w49) -> (.not. x?=w53:bool)
        n10 = Not(x=w48) -> (.not. x?=w52:bool)
        n11 = Build Array(w52, w53) -> (w50:bool[])
        n12 = call-poly <vilib>:"DAQmx Write.vi"("task/channels in"=w51, "data"=w50, "error in"=w47) -> ("error out"=w45:errorcluster)  [unwired: 10 in, 2 out]
      }
    }
    n13 = call <vilib>:"General Error Handler.vi"("error in (no error)"=w40) -> ()  [unwired: 10 in, 5 out]
  }
  n14 = property on="Acquire Time" class="DigNum (strict)"() -> ("Value"=w2:i32)  [unwired: 2 in, 2 out]
  n15 = property on="DAQ Settings" class="Clust (strict)"() -> ("Value"=w5:T13)  [unwired: 2 in, 2 out]
  n16 = control-ref of="Run Options"() -> (w17:refnum<vi>)
  n17 = Unbundle By Name(w5) -> ("Rate"=w7:dbl, "Shutter Task"=w10:refnum<k21>)
  n18 = control-ref of="Counts per image"() -> (w30:refnum<vi>)
  n19 = control-ref of="Count Rate / s"() -> (w13:refnum<vi>)
  n20 = control-ref of="Bakc Image"() -> (w25:refnum<vi>)
  n21 = control-ref of="Centroiding"() -> (w26:refnum<vi>)
  n22 = property on="Scan Set up" class="Clust (strict)" props=["Value"]() -> ()  [unwired: 2 in, 3 out]
  n23 = Multiply(x=w2, y=w7) -> (x*y=w6:dbl)
  n24 = control-ref of="Collection Results"() -> (w32:refnum<vi>)
  n25 = control-ref of="Current Image"() -> (w29:refnum<vi>)
  n26 = control-ref of="Image Options"() -> (w27:refnum<vi>)
  n27 = Bundle By Name(cluster=w5, "Number of Samples"=w6) -> (w8:T13)
  n28 = control-ref of="Bakc Image2"() -> (w24:refnum<vi>)
  n29 = control-ref of="Stop Collect"() -> (w33:refnum<vi>)
  n30 = control-ref of="Information"() -> (w31:refnum<vi>)
  n31 = control-ref of="Signal Image"() -> (w23:refnum<vi>)
  n32 = Current VI's Path() -> (path=w22:path)
  n33 = Not A Number/Path/Refnum?(number/path/refnum=w10) -> (NaN/Path/Refnum?=w9:bool)
  n34 = case shown="True" w9 {
    tunnel: w8 -> [w54 w57]
    tunnel: "Error In" -> [w56 w58]
    tunnel: [w55 w58] -> w12
    tunnel: [w54 w57] -> w11
    frame False {
      n35 = call "DAQ_clean_daq.vi"("Error In"=w56, "DAQ Settings"=w54) -> ("Error Out"=w55:errorcluster)  [unwired: 3 in]
    }
    frame True {
    }
  }
  n36 = Bundle By Name(cluster="Ref Cluster 1", "Stop Collect"=w33, "Collection Information"=w32, "Infromation"=w31, "Counts per image"=w30, "Image Control Reference"=w29, "Run Options"=w17, "Image Options"=w27, "Centroiding"=w26, "Image"=w23, "Bakc Image"=w25, "Bakc Image 2"=w24, "Count Rate / s"=w13) -> (w28:T2)
  n37 = Build Path(base path=w22, name or relative path=path "..") -> (appended path=w19:path)
  n38 = Build Path(base path=w19, name or relative path="mcp_hit_test.png") -> (appended path=w18:path)
  n39 = property on="Test Image File Path" class="Path"(error in="Error In", "Value"=w18) -> ()  [unwired: 1 in, 2 out]
  n40 = call "DAQ_set_all.vi"("Error In"=w12, "DAQ Settings"=w11) -> ("Error Out"=w3:errorcluster, "DAQ Out"=w4:T13)  [unwired: 2 in]
  n41 = property on="Collect" class="Bool (strict)"(error in="Error In", "DisabledEnum"=w37) -> (error out=w16:errorcluster)  [unwired: 1 in, 1 out]
  n42 = property on="Moving" class="Bool (strict)"("Blinking"=w14) -> ()  [unwired: 2 in, 2 out]
  n43 = property on="Setup?" class="Bool (strict)"("Blinking"=w14) -> ()  [unwired: 2 in, 2 out]
  n44 = property on="Running" class="Bool (strict)"("Value"=w14) -> ()  [unwired: 2 in, 2 out]
  n45 = property on="Delay Moving" class="Bool (strict)"("Blinking"=w14) -> ()  [unwired: 2 in, 2 out]
  n46 = property on="DAQ Settings" class="Clust (strict)"(error in=w3, "Value"=w4) -> ()  [unwired: 1 in, 2 out]
  n47 = property on="Scan Type" class="Ring (strict)"(error in=w16, "Val(Sgnl)"=u16 0 ("Value")) -> ()  [unwired: 1 in, 2 out]
  n48 = property on="Stop Collect" class="Bool (strict)"(error in=w16, "DisabledEnum"=w37) -> (error out=w36:errorcluster)  [unwired: 1 in, 1 out]
  n49 = while {
    shift-right: [w62] -> w38
    shift-left: w36 -> [w61]
    tunnel: w28 -> [w59]
    stop <- w60 stop-if-true
    n50 = event shown="[2] \"New Collect\": Value Change" {
      selector: _ -> [_ _ _ _ _ _ _ _ _ _]
      dyn-events: _ -> [_ _ _ _ _ _ _ _ _ _]
      timeout: _ -> [_ _ _ _ _ _ _ _ _ _]
      tunnel: [w64 w73 w103 w439 w516 w580 w699 w721 w738 w753] -> w62
      tunnel: w61 -> [w64 w92 w99 w430 w518 w581 w697 w723 w747 w757]
      tunnel: [FALSE FALSE _ FALSE FALSE _ FALSE FALSE TRUE _] -> w60
      tunnel: w59 -> [_ w80 w100 _ _ _ _ _ _ _]
      event Timeout {
        n51 = event-data() -> ()  [unwired: 1 in, 3 out]
      }
      event "Collect": Value Change {
        w81 = FALSE ("Collect")
        # "Replaced Image type"
        n52 = event-data() -> ()  [unwired: 1 in, 6 out]
        n53 = property on="Collection Information" class="Arr (strict)"() -> ("Value"=w77:T10[])  [unwired: 2 in, 2 out]
        n54 = property on="Stop Collect" class="Bool (strict)"(error in=w92, "DisabledEnum"=T18."Enabled" ("Disabled")) -> ()  [unwired: 1 in, 2 out]
        n55 = property on="Queue Check" class="Bool (strict)" props=["Value"]() -> ()  [unwired: 2 in, 3 out]
        n56 = property on="Big_image Array" class="Arr (strict)"() -> ("Value"=w75:i16[][][])  [unwired: 2 in, 2 out]
        n57 = property on="Image types Bool" class="Arr (strict)"() -> ("Value"=w85:bool[])  [unwired: 2 in, 2 out]
        n58 = property on="Camera Set" class="IMAQImage (strict)"() -> ("Value"=w86:T5)  [unwired: 2 in, 2 out]
        n59 = property on="Queue Array" class="Arr (strict)"() -> ("Value"=w84:T4[])  [unwired: 2 in, 2 out]
        n60 = property on="Session Out" class="IMAQdx (strict)"() -> ("Value"=w72:T3)  [unwired: 2 in, 2 out]
        n61 = property on="Peak Find Settings" class="Clust (strict)"() -> ("Value"=w74:T23)  [unwired: 2 in, 2 out]
        n62 = call "VMI_acquire_subV_Arrays.vi"("Big_image Array"=w75, "Queue Array"=w84, "IMAQ In"=w86, "error in (no error)"=w92, "Types to acquire in"=w85, "Collection Information"=w77, "Peak Find Settings"=w74, "Session Out"=w72, "Ref Cluster 1"=w80) -> ("Points per image"=→"Points per image":i32[], "Histogram_array"=w65:i32[][], "Signal Background"=w68:cluster{"X":sgl, "Y":sgl}[], "Background"=w67:cluster{"X":sgl, "Y":sgl}[], "Background 2"=w66:cluster{"X":sgl, "Y":sgl}[], "error out"=w69:errorcluster)  [unwired: 4 in, 1 out]
        n63 = Array Size(array=w66) -> (size(s)=→"size(s) 3":i32)
        n64 = Array Size(array=w67) -> (size(s)=→"size(s) 2":i32)
        n65 = property on="Background 1" class="Arr (strict)"("Value"=w67) -> ()  [unwired: 2 in, 2 out]
        n66 = property on="Signal Background" class="Arr (strict)"("Value"=w68) -> ()  [unwired: 2 in, 2 out]
        n67 = property on="Background 2" class="Arr (strict)"("Value"=w66) -> ()  [unwired: 2 in, 2 out]
        n68 = Array Size(array=w68) -> (size(s)=→"size(s)":i32)
        n69 = property on="Histogram_array" class="Arr (strict)"("Value"=w65) -> ()  [unwired: 2 in, 2 out]
        n70 = property on="Camera Settings" class="Clust (strict)"(error in=w69) -> ("Value"=w76:T16)  [unwired: 1 in, 2 out]
        n71 = Unbundle By Name(w76) -> ("Run Options"=w71:u16)
        n72 = call "VMI_clean_up_Camera.vi"("Error In"=w69, "Run Options"=w71, "Camera Session"=w72) -> ("Error Out"=w70:errorcluster)  [unwired: 4 in]
        n73 = property on="Signal Image" class="Arr (strict)"(error in=w69) -> ("Value"=w79:i16[][])  [unwired: 1 in, 2 out]
        n74 = Array Max & Min(array=w79) -> (max value=→"max value":i16)  [unwired: 3 out]
        n75 = property on="Collect" class="Bool (strict)"(error in=w69, "Value"=w81) -> ()  [unwired: 1 in, 2 out]
        n76 = property on="Stop Collect" class="Bool (strict)"(error in=w69, "DisabledEnum"=T18."Disabled and Grayed Out" ("Disabled"), "Value"=w81) -> (error out=w91:errorcluster)  [unwired: 1 in, 1 out]
        n77 = Merge Errors(w91, w70) -> (w73:errorcluster)
      }
      event "New Collect": Value Change {
        w95 = "https://hooks.slack.com/services/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" ("Slack Webhook")
        w102 = FALSE ("Stop Collect")
        # "Collect Images using new collection subVIs"
        n78 = event-data() -> ()  [unwired: 1 in, 6 out]
        n79 = property on="Delay Scan?" class="Bool (strict)"(error in=w99) -> ("Value"=w106:bool)  [unwired: 1 in, 2 out]
        n80 = property on="Peak Find Settings" class="Clust (strict)"(error in=w99) -> ("Value"=w114:T23)  [unwired: 1 in, 2 out]
        n81 = property on="Session Out" class="IMAQdx (strict)"(error in=w99) -> ("Value"=w105:T3)  [unwired: 1 in, 2 out]
        n82 = property on="Queue Array" class="Arr (strict)"(error in=w99) -> ("Value"=w118:T4[])  [unwired: 1 in, 2 out]
        n83 = property on="Running" class="Bool (strict)"(error in=w99, "Value"=TRUE ("Running")) -> ()  [unwired: 1 in, 2 out]
        n84 = property on="Big_image Array" class="Arr (strict)"(error in=w99) -> ("Value"=w115:i16[][][])  [unwired: 1 in, 2 out]
        n85 = property on="Collection Information" class="Arr (strict)"(error in=w99) -> ("Value"=w94:T10[])  [unwired: 1 in, 2 out]
        n86 = property on="Image Set" class="IMAQImage (strict)"(error in=w99) -> ("Value"=w109:T5)  [unwired: 1 in, 2 out]
        n87 = property on="Stop Collect" class="Bool (strict)"(error in=w99, "DisabledEnum"=T18."Enabled" ("Disabled")) -> ()  [unwired: 1 in, 2 out]
        n88 = property on="Information" class="Str"(error in=w99, "Value"="Collecting" ("Information")) -> ()  [unwired: 1 in, 2 out]
        n89 = property on="AI Task" class="DAQmxName (strict)"() -> ("Value"=w108:refnum<k21>)  [unwired: 2 in, 2 out]
        n90 = property on="Shutter Task" class="DAQmxName (strict)"() -> ("Value"=w107:refnum<k21>)  [unwired: 2 in, 2 out]
        n91 = Bundle By Name(cluster=T19 {"IMAQ In"=refnum, "Camera Session"="", "Shutter Task"="", "AI task"=""} ("IO settings"), "IMAQ In"=w109, "Camera Session"=w105, "Shutter Task"=w107, "AI task"=w108) -> (w110:T19)
        n92 = case shown="True" w106 {
          tunnel: w100 -> [w145 w162]
          tunnel: w118 -> [w144 w165]
          tunnel: w94 -> [w139 w155]
          tunnel: w115 -> [w143 w161]
          tunnel: w114 -> [w142 w164]
          tunnel: w99 -> [w141 w151]
          tunnel: [w129 w159] -> w96
          tunnel: w110 -> [w140 w163]
          tunnel: w100 -> [_ w156]
          tunnel: w95 -> [_ w153]
          frame False {
            # "Just image no delay"
            n93 = call "VMI_acquire_rewrite_v2.vi"("IO settings"=w140, "Queue Array"=w144, "Peak Find Settings"=w142, "Collection Information"=w139, "error in"=w141, "Ref Cluster 1"=w145, "Big_image Array"=w143) -> ("Histogram"=w133:i32[][], "Peak Array"=w137:cluster{"X":sgl, "Y":sgl}[][], "Powers"=w136:dbl[][], "Power Err"=w135:dbl[][], "xaxis"=w132:i32[][], "error IO"=w129:errorcluster)  [unwired: 2 in, 1 out]
            "Peak Array" <- w137
            "AI in" <- w136
            "AI err" <- w135
            "Histogram_array" <- w133
            n94 = property on="Peaks" class="Arr (strict)"() -> ("Value"=w131:T1[])  [unwired: 2 in, 2 out]
            n95 = Array Size(array=w139) -> (size(s)=w138:i32)
            n96 = call "VMI_data_sort.vi"("Power Err"=w135, "Numeric"=w138, "xaxis"=w132, "Histogram"=w133, "Powers"=w136, "Peak Array"=w137, "Data"=w131) -> ("Data Out"=w130:T1[], "HistArray"=→"Hist_full":dbl[][][])  [unwired: 3 in]
            n97 = property on="Peaks" class="Arr (strict)"("Value"=w130) -> ()  [unwired: 2 in, 2 out]
          }
          frame True {
            # "Delay scan"
            n98 = control-ref of="CmdStopDelay"() -> (w157:refnum<vi>)
            n99 = control-ref of="Postion / mm"() -> (w158:refnum<vi>)
            n100 = property on="Backup Path" class="Path"() -> ("Value"=w146:path)  [unwired: 2 in, 2 out]
            n101 = property on="Delay Cluster" class="Clust (strict)"(error in=w151) -> ("Value"=w152:T11)  [unwired: 1 in, 2 out]
            n102 = property on="Accurate Scan" class="Bool (strict)"(error in=w151) -> (error out=w160:errorcluster, "Value"=w166:bool)  [unwired: 1 in, 1 out]
            n103 = property on="Main Directory" class="Path"() -> ("Value"=w154:path)  [unwired: 2 in, 2 out]
            n104 = Unbundle By Name(w152) -> ("Delay List"=w147:string[][], "Conn. Axes"=w150:string[], "System no."=w149:i32, "Stage Number"=w148:i32)
            n105 = case shown="False" w166 {
              tunnel: w160 -> [w170 w280]
              tunnel: w165 -> [w202 w310]
              tunnel: w164 -> [w203 w309]
              tunnel: w163 -> [w204 w308]
              tunnel: w155 -> [w190 w285]
              tunnel: w162 -> [w201 w307]
              tunnel: w161 -> [w200 w306]
              tunnel: [w168 w302] -> w159
              tunnel: w157 -> [w196 w300]
              tunnel: w158 -> [w199 w301]
              tunnel: w156 -> [_ _]
              tunnel: w154 -> [_ w299]
              tunnel: w153 -> [_ w294]
              tunnel: w152 -> [w173 w283]
              tunnel: w150 -> [w179 _]
              tunnel: w149 -> [w178 _]
              tunnel: w149 -> [w177 _]
              tunnel: w148 -> [w176 _]
              tunnel: w147 -> [_ w278]
              tunnel: w146 -> [_ w277]
              frame False {
                w174 = i32[] []
                w175 = TRUE ("Blinking")
                w186 = 1.0 ("Relative Integration Time")
                w167 = FALSE ("Blinking")
                # "Check collection\nsettings are good for delays"
                # "Collect while moving - only need counts"
                n106 = property on="Scan End / mm" class="DigNum (strict)"() -> ("Value"=w171:dbl)  [unwired: 2 in, 2 out]
                n107 = property on="Collection Results" class="Clust (strict)"(error in=w170) -> ("Value"=w185:T7)  [unwired: 1 in, 2 out]
                n108 = Bundle By Name(cluster=w173, "Target Position / mm"=w171) -> (w172:T11)
                n109 = property on="Scan Start /mm" class="DigNum (strict)"(error in=w170) -> ("Value"=w182:dbl)  [unwired: 1 in, 2 out]
                n110 = property on="Moving" class="Bool (strict)"(error in=w170, "Blinking"=w175) -> ()  [unwired: 1 in, 2 out]
                n111 = property on="Delay Moving" class="Bool (strict)"(error in=w170, "Value"=w175) -> ()  [unwired: 1 in, 2 out]
                n112 = call "Scans_move_1_delay.vi"("Target Offset / mm"=-0.1, "Error In"=w170, "Target Position / mm"=w182, "Repeat Velocity / mms-1"=3.0, "Delay Cluster"=w173) -> ("error out"=w169:errorcluster)  [unwired: 6 in]
                n113 = call "VMI_set_delay_times.vi"("Collection Constant In"=w185, "Error In"=w170, "Relative Integration Time"=w186, "Base Integration Time"=w186) -> ("Error Out"=w183:errorcluster, "Collection Constant Out"=w184:T7)  [unwired: 6 in]
                n114 = call "VMI_move_wait_PI.vi"("SetV?"=TRUE, "Move and Wait?"=FALSE, "Delay Cluster"=w172, "Error In"=w169, "Stop ref"=w196, "Postion / mm"=w199) -> ("error out"=w188:errorcluster)  [unwired: 5 in]
                n115 = property on="Collection Results" class="Clust (strict)"(error in=w183, "Value"=w184) -> ()  [unwired: 1 in, 2 out]
                n116 = Merge Errors(w183, w188) -> (w187:errorcluster)
                n117 = while {
                  tunnel: w204 -> [w256]
                  tunnel: w203 -> [w255]
                  tunnel: w202 -> [w254]
                  tunnel: w190 -> [w253]
                  tunnel: w201 -> [w252]
                  tunnel: w200 -> [w251]
                  shift-right: [w213] -> w168
                  shift-left: w187 -> [w250]
                  tunnel: w196 -> [w246]
                  shift-right: [w235] -> w195
                  shift-left: w174 -> [w237]
                  shift-right: [w233] -> w194
                  shift-left: w174 -> [w236]
                  shift-right: [w226] -> w193
                  shift-left: _ -> [w225]
                  shift-right: [w221] -> w192
                  shift-left: _ -> [w220]
                  tunnel: w179 -> [w217]
                  tunnel: w178 -> [w216]
                  tunnel: w177 -> [w215]
                  tunnel: w176 -> [w214]
                  i -> [w241]
                  stop <- w212 stop-if-true
                  w224 = 0 ("index (row)")
                  w229 = 0 ("index (row)")
                  w228 = 0 ("index (row)")
                  n118 = call "VMI_acquire_rewrite_v2.vi"("IO settings"=w256, "Queue Array"=w254, "Peak Find Settings"=w255, "Collection Information"=w253, "error in"=w250, "Ref Cluster 1"=w252, "Big_image Array"=w251) -> ("Histogram"=w240:i32[][], "Powers"=w230:dbl[][], "Power Err"=w223:dbl[][], "error IO"=w249:errorcluster)  [unwired: 2 in, 3 out]
                  n119 = call "#5.vi"("System no."=w216, "error in"=w249) -> ("Axis moving?"=w248:bool[], "error out"=w247:errorcluster)  [unwired: 16 in]
                  n120 = call "POS?.vi"("System no."=w215, "Axes to query"=w217, "error in"=w247) -> ("Position"=w219:dbl[], "error out"=w213:errorcluster)  [unwired: 15 in]
                  n121 = Index Array(array=w223, index (row)=w224, index (col)=w224) -> (element=w222:dbl)
                  n122 = Index Array(array=w230, index (row)=w229, index (col)=w229) -> (element=w227:dbl)
                  n123 = Index Array(array=w219, index=0) -> (element=w218:dbl)
                  n124 = Index Array(array=w240, index (row)=w228, index (col)=w228) -> (element=w238:i32)
                  n125 = property class="Bool (strict)"(reference=w246) -> ("Value"=w245:bool)  [unwired: 1 in, 2 out]
                  n126 = Equal To 0?(x=w241) -> (x = 0?=w239:bool)
                  n127 = case shown="False" w239 {
                    tunnel: w238 -> [w264 w274]
                    tunnel: w218 -> [w267 w276]
                    tunnel: [w266 w275] -> w235
                    tunnel: w237 -> [w268 _]
                    tunnel: [w263 w273] -> w233
                    tunnel: w236 -> [w265 _]
                    tunnel: w227 -> [w261 w272]
                    tunnel: [w260 w271] -> w226
                    tunnel: w225 -> [w262 _]
                    tunnel: w222 -> [w258 w270]
                    tunnel: [w257 w269] -> w221
                    tunnel: w220 -> [w259 _]
                    frame False {
                      n128 = Build Array (concatenate)(w259, w258) -> (w257:dbl[])
                      n129 = Build Array (concatenate)(w268, w267) -> (w266:dbl[])
                      n130 = Build Array (concatenate)(w262, w261) -> (w260:dbl[])
                      n131 = Build Array (concatenate)(w265, w264) -> (w263:i32[])
                    }
                    frame True {
                      n132 = Build Array(w272) -> (w271:dbl[])
                      n133 = Build Array(w270) -> (w269:dbl[])
                      n134 = Build Array(w274) -> (w273:i32[])
                      n135 = Build Array(w276) -> (w275:dbl[])
                    }
                  }
                  n136 = Index Array(array=w248, index=w214) -> (element=w243:bool)
                  n137 = Not(x=w243) -> (.not. x?=w211:bool)
                  n138 = Or(x=w245, y=w211) -> (x .or. y?=w244:bool)
                  n139 = property on="Postion / mm" class="Arr (strict)"("Value"=w219) -> ()  [unwired: 2 in, 2 out]
                  n140 = call "Convert to Dynamic Data"("Array"=w235) -> ("Dynamic Data Type"=w234:dynamicdata)  [unwired: 3 in]
                  n141 = call "Convert to Dynamic Data2"("Array"=w233) -> ("Dynamic Data Type"=w232:dynamicdata)  [unwired: 3 in]
                  n142 = call "Build XY Graph"("Y Input"=w232, "X Input"=w234) -> ("XY Graph"=w231:cluster{"X":dbl[], "Y":dbl[]}[])  [unwired: 8 in, 1 out]
                  n143 = property on="Stop Collect" class="Bool (strict)"(error in=w213) -> ("Value"=w210:bool)  [unwired: 1 in, 2 out]
                  n144 = property on="Stage Position" class="DigNum (strict)"("Value"=w218) -> ()  [unwired: 2 in, 2 out]
                  n145 = Or(x=w210, y=w244) -> (x .or. y?=w212:bool)
                  n146 = property on="Counts per image" class="XYGraph (strict)"("Value"=w231) -> ()  [unwired: 2 in, 2 out]
                }
                n147 = Array Size(array=w190) -> (size(s)=w189:i32)
                n148 = for {
                  N: w189 -> [_]
                  tunnel: w194 -> [w209]
                  tunnel: w193 -> [w208]
                  tunnel: w192 -> [w207]
                  tunnel: [w206] -> w191 mode=indexing
                  tunnel: w195 -> [w205]
                  n149 = Build Array(w205, w209, w208, w207) -> (w206:dbl[][])
                }
                n150 = property on="Moving" class="Bool (strict)"(error in=w168, "Blinking"=w167) -> ()  [unwired: 1 in, 2 out]
                n151 = property on="Delay Moving" class="Bool (strict)"(error in=w168, "Value"=w167) -> ()  [unwired: 1 in, 2 out]
                n152 = property on="Hist_full" class="Arr (strict)"(error in=w168, "Value"=w191) -> ()  [unwired: 1 in, 2 out]
              }
              frame True {
                w293 = dbl[][][] []
                # "Move then collect get image at each point"
                n153 = Index Array(array=w285, index=0) -> (element=w287:T10)
                n154 = Unbundle By Name(w287) -> ("LaserWave1"=w289:dbl, "LaserWave2"=w288:dbl)
                n155 = call "VMI_set_delay_list.vi"("Table"=w278, "Pump"=w289, "Probe"=w288) -> ("Number delays"=w292:i32, "Delay_list"=w291:dbl[][], "Delay_full_dir"=w290:string[], "First Point"=w284:dbl)  [unwired: 1 out]
                "Delay Scan Steps" <- w292
                n156 = property on="Delay" class="Slide (strict)"("Scale.Maximum"=w292) -> ()  [unwired: 2 in, 2 out]
                n157 = call "Scans_move_1_delay.vi"("Target Offset / mm"=-0.1, "Error In"=w280, "Target Position / mm"=w284, "Repeat Velocity / mms-1"=3.0, "Delay Cluster"=w283) -> ("error out"=w279:errorcluster)  [unwired: 6 in]
                n158 = call "VMI_save_delay_paths.vi"("error in"=w280, "Remote path 2"=w277, "Delay_full_dir"=w290, "Main Directory"=w299) -> ("appended path"=w295:path, "Delay_paths"=w297:path[], "New Date Name"=w298:string)  [unwired: 1 out]
                n159 = property on="Save Path" class="Path"("Value"=w295) -> ()  [unwired: 2 in, 2 out]
                n160 = property on="Current File Date and endings" class="Str"("Value"=w298) -> ()  [unwired: 2 in, 2 out]
                n161 = while {
                  tunnel: w310 -> [w367]
                  tunnel: w309 -> [w366]
                  tunnel: w308 -> [w365]
                  tunnel: w285 -> [w329]
                  tunnel: w307 -> [w364]
                  tunnel: w306 -> [w363]
                  tunnel: w292 -> [w335]
                  tunnel: w291 -> [w362]
                  tunnel: w300 -> [w358]
                  tunnel: w301 -> [w361]
                  tunnel: TRUE ("Move and Wait?") -> [w360]
                  tunnel: FALSE ("SetV?") -> [w359]
                  shift-right: [w337] -> w302
                  shift-left: w279 -> [w315]
                  shift-right: [w332] -> _
                  shift-left: w293 -> [w346]
                  shift-right: [w334] -> _
                  shift-left: cluster{"X":sgl, "Y":sgl}[][][] [] ("Peak Array") -> [w348]
                  shift-right: [w333] -> _
                  shift-left: w293 -> [w345]
                  shift-right: [w331] -> _
                  shift-left: w293 -> [w343]
                  tunnel: w284 -> [_]
                  shift-right: [w330] -> _
                  shift-left: _ -> [w351]
                  tunnel: w297 -> [w327]
                  tunnel: w294 -> [w322]
                  i -> [w319]
                  stop <- w326 stop-if-true
                  n162 = Quotient & Remainder(x=w319, y="Loops per Save") -> (x-y*floor(x/y)=w339:i32)  [unwired: 1 out]
                  n163 = for {
                    N: w335 -> [_]
                    tunnel: w367 -> [w427]
                    tunnel: w366 -> [w426]
                    tunnel: w365 -> [w425]
                    tunnel: w329 -> [w424]
                    tunnel: w364 -> [w423]
                    tunnel: w363 -> [w422]
                    shift-right: [w421] -> w338
                    shift-left: w315 -> [w401]
                    tunnel: w362 -> [w418] mode=indexing
                    tunnel: w358 -> [w414]
                    tunnel: w361 -> [w413]
                    tunnel: w360 -> [w412]
                    tunnel: w359 -> [w411]
                    tunnel: [w410] -> w347 mode=indexing
                    tunnel: [w409] -> w349 mode=indexing
                    tunnel: [w408] -> w344 mode=indexing
                    tunnel: [w407] -> w342 mode=indexing
                    tunnel: w319 -> [w391]
                    tunnel: [w391] -> w352 mode=indexing
                    tunnel: [w390] -> _
                    i -> [w392]
                    # "This loop will move across each delay in turn and collect images"
                    n164 = Index Array(array=w418, index #1=1 ("index"), index #2=2 ("index")) -> (element #1=w417:dbl, element #2=w403:dbl)
                    n165 = property on="Collection Results" class="Clust (strict)"(error in=w401) -> (error out=w399:errorcluster, "Value"=w402:T7)  [unwired: 1 in, 1 out]
                    n166 = property on="Target Position / mm" class="DigNum (strict)"(error in=w401, "Value"=w417) -> (error out=w420:errorcluster)  [unwired: 1 in, 1 out]
                    n167 = property on="Delay Cluster" class="Clust (strict)"(error in=w420) -> (error out=w419:errorcluster, "Value"=w398:T11)  [unwired: 1 in, 1 out]
                    n168 = call "VMI_set_delay_times.vi"("Collection Constant In"=w402, "Error In"=w401, "Relative Integration Time"=w403, "Base Integration Time"=1.0) -> ("Error Out"=w405:errorcluster, "Collection Constant Out"=w400:T7)  [unwired: 6 in]
                    n169 = call "VMI_move_wait_PI.vi"("SetV?"=w411, "Move and Wait?"=w412, "Delay Cluster"=w398, "Error In"=w419, "Stop ref"=w414, "Postion / mm"=w413) -> ("error out"=w390:errorcluster)  [unwired: 5 in]
                    n170 = Unbundle By Name(w398) -> ("System no."=w397:i32, "Conn. Axes"=w396:string[])
                    n171 = property on="Collection Results" class="Clust (strict)"(error in=w399, "Value"=w400) -> ()  [unwired: 1 in, 2 out]
                    n172 = Merge Errors(w405, w390) -> (w406:errorcluster)
                    n173 = call "POS?.vi"("System no."=w397, "Axes to query"=w396, "error in"=w390) -> ("Position"=w395:dbl[])  [unwired: 15 in, 1 out]
                    n174 = call "VMI_acquire_rewrite_v2.vi"("IO settings"=w425, "Queue Array"=w427, "Peak Find Settings"=w426, "Collection Information"=w424, "error in"=w406, "Ref Cluster 1"=w423, "Big_image Array"=w422) -> ("Histogram"=w410:i32[][], "Peak Array"=w409:cluster{"X":sgl, "Y":sgl}[][], "Powers"=w408:dbl[][], "Power Err"=w407:dbl[][], "error IO"=w421:errorcluster)  [unwired: 2 in, 2 out]
                    n175 = Index Array(array=w395, index=0) -> (element=w393:dbl)
                    n176 = property on="Postion / mm" class="Arr (strict)"("Value"=w395) -> ()  [unwired: 2 in, 2 out]
                    n177 = property on="Stage Position" class="DigNum (strict)"("Value"=w393) -> ()  [unwired: 2 in, 2 out]
                    "Delay Loop" <- w392
                    "Delay" <- w392
                  }
                  n178 = Equal To 0?(x=w339) -> (x = 0?=w340:bool)
                  n179 = property on="Auto Save" class="Bool (strict)"() -> ("Value"=w328:bool)  [unwired: 2 in, 2 out]
                  n180 = And(x=w328, y=w340) -> (x .and. y?=w325:bool)
                  n181 = property class="Bool (strict)"(reference=w358, error in=w338) -> (error out=w316:errorcluster, "Value"=w357:bool)  [unwired: 1 out]
                  n182 = Build Array (concatenate)(w351, w352) -> (w330:i32[][])
                  n183 = property on="Stop Collect" class="Bool (strict)"(error in=w338) -> ("Value"=w356:bool)  [unwired: 1 in, 2 out]
                  n184 = Or(x=w357, y=w356) -> (x .or. y?=w326:bool)
                  n185 = Or(x=w325, y=w326) -> (x .or. y?=w324:bool)
                  n186 = Index Array(array=w347, index (dim 1)=0 ("index (page)")) -> (element=w354:i32[][])  [unwired: 2 in]
                  n187 = call "VMI_delays_combine.vi"("Peak Array All"=w348, "AI per delay All"=w345, "Peak Array Current"=w349, "AI per delay Current"=w344, "Delay Number"=w335, "Counts per delay All"=w346, "Std per delay All"=w343, "Counts per delay Current"=w347, "Std per delay Current"=w342) -> ("Peak Out"=w334:cluster{"X":sgl, "Y":sgl}[][][], "AI Out"=w333:dbl[][][], "Counts Out"=w332:dbl[][][], "Std Out"=w331:dbl[][][])  [unwired: 3 in]
                  n188 = case shown="True" w324 {
                    tunnel: w338 -> [w371 w389]
                    tunnel: [w371 w388] -> w337
                    tunnel: w335 -> [_ w387]
                    tunnel: w334 -> [_ w384]
                    tunnel: w333 -> [_ w383]
                    tunnel: w332 -> [_ w382]
                    tunnel: w331 -> [_ w381]
                    tunnel: w330 -> [_ w380]
                    tunnel: w329 -> [_ w377]
                    tunnel: w327 -> [_ w372]
                    frame False {
                    }
                    frame True {
                      n189 = property on="Current File Date and endings" class="Str"() -> ("Value"=w373:string)  [unwired: 2 in, 2 out]
                      n190 = property on="Image Info Acqu" class="Clust (strict)"() -> ("Value"=w375:T8)  [unwired: 2 in, 2 out]
                      n191 = property on="Files to Save" class="Arr (strict)"() -> ("Value"=w374:bool[])  [unwired: 2 in, 2 out]
                      n192 = Bundle By Name(cluster=T21 {"Peak Array All"=[], "AI per delay All"=[], "Counts per delay All"=[], "Std per delay All"=[], "Hit x"=[]} ("Results"), "Peak Array All"=w384, "AI per delay All"=w383, "Counts per delay All"=w382, "Std per delay All"=w381, "Hit x"=w380) -> (w385:T21)
                      n193 = Bundle By Name(cluster=T20 {"Collection Information"=[], "ChangeFile"=FALSE, "Image Info"={"X size"=782.0, "Y size"=582.0, "Centroiding"=1.0}, "SAve Paths"=[], "Save"=[], "Current File Date"=""} ("Save Info"), "Collection Information"=w377, "ChangeFile"=FALSE, "Image Info"=w375, "SAve Paths"=w372, "Save"=w374, "Current File Date"=w373) -> (w378:T20)
                      n194 = call "VMI_delays_save_display.vi"("error in"=w389, "Save Info"=w378, "Results"=w385, "Delay Number"=w387) -> ("error out"=w388:errorcluster)  [unwired: 2 in]
                    }
                  }
                  n195 = Number To Decimal String(number=w319) -> (decimal integer string=w320:string)  [unwired: 1 in]
                  n196 = call "Convert to Dynamic Data4"("2D Array"=w330) -> ("Dynamic Data Type"=w350:dynamicdata)  [unwired: 3 in]
                  n197 = call "Convert to Dynamic Data3"("2D Array"=w354) -> ("Dynamic Data Type"=w353:dynamicdata)  [unwired: 3 in]
                  n198 = property on="Slack" class="Bool (strict)"(error in=w316) -> ("Value"=w323:bool)  [unwired: 1 in, 2 out]
                  n199 = Concatenate Strings("Delay scan ", w320, " done" ("string")) -> (w317:string)
                  n200 = call "Build Delay Graph"("Y Input"=w353, "X Input"=w350) -> ("XY Graph"=w355:cluster{"X":dbl[], "Y":dbl[]}[])  [unwired: 8 in, 1 out]
                  n201 = case shown="True" w323 {
                    tunnel: w322 -> [_ w370]
                    tunnel: w317 -> [_ w368]
                    frame False {
                    }
                    frame True {
                      n202 = call "Slack_HTTP_POST.vi"("Info String"=w368, "Slack Webhook"=w370) -> ("Sent string"=w369:string)  [unwired: 1 in, 1 out]
                      n203 = property on="Last Slack" class="Str"("Value"=w369) -> ()  [unwired: 2 in, 2 out]
                    }
                  }
                  n204 = property on="Counts per image" class="XYGraph (strict)"("Value"=w355) -> ()  [unwired: 2 in, 2 out]
                  "Total Loop" <- w319
                }
                n205 = property on="Log File" class="Bool (strict)"(error in=w279) -> ("Value"=w296:bool)  [unwired: 1 in, 2 out]
                n206 = case shown="True" w296 {
                  tunnel: w295 -> [_ w312]
                  tunnel: w285 -> [_ w311]
                  frame False {
                  }
                  frame True {
                    n207 = property on="Delay Cluster" class="Clust (strict)"() -> ("Value"=w313:T11)  [unwired: 2 in, 2 out]
                    n208 = property on="Scan Set up" class="Clust (strict)"() -> ("Value"=w314:T9)  [unwired: 2 in, 2 out]
                    n209 = call "Scan_ctrl.vi"("Scan Set up"=w314, "appended path"=w312, "Value"=w311, "Delay Cluster"=w313) -> ()  [unwired: 3 in, 2 out]
                  }
                }
              }
            }
          }
        }
        n210 = case shown="True" "Slack" {
          tunnel: w99 -> [_ w121]
          tunnel: w94 -> [_ w128]
          tunnel: w95 -> [_ w119]
          frame False {
          }
          frame True {
            n211 = property on="Scan Set up" class="Clust (strict)"(error in=w121) -> (error out=w120:errorcluster, "Value"=w126:T9)  [unwired: 1 in, 1 out]
            n212 = property on="Scan Type" class="Ring (strict)"() -> ("RingText.Text"=w124:string)  [unwired: 2 in, 2 out]
            n213 = property on="Current File Date and endings" class="Str"() -> ("Value"=w127:string)  [unwired: 2 in, 2 out]
            n214 = Unbundle By Name(w126) -> ("Chemical"=w125:string)
            n215 = call "Build_Slack_text.vi"("Collection Info Array"=w128, "Chemical"=w125, "Scan Type"=w124, "New Date Name"=w127) -> ("Slack String"=w123:string)  [unwired: 7 in]
            n216 = call "Slack_HTTP_POST.vi"("error in (no error)"=w120, "Info String"=w123, "Slack Webhook"=w119) -> ("Sent string"=→"Last Slack":string)  [unwired: 1 out]
          }
        }
        n217 = property on="Run Options" class="Ring (strict)"(error in=w96) -> ("Value"=w112:u16)  [unwired: 1 in, 2 out]
        n218 = call "VMI_clean_up_Camera.vi"("Error In"=w96, "Run Options"=w112, "Camera Session"=w105) -> ("Error Out"=w113:errorcluster)  [unwired: 4 in]
        n219 = property on="Information" class="Str"(error in=w96, "Value"="Finished Collecting" ("Information")) -> ()  [unwired: 1 in, 2 out]
        n220 = Merge Errors(w96, w113) -> (w103:errorcluster)
        n221 = property on="Stop Collect" class="Bool (strict)"(error in=w103, "DisabledEnum"=T18."Disabled and Grayed Out" ("Disabled"), "Value"=w102) -> ()  [unwired: 1 in, 2 out]
        n222 = property on="New Collect" class="Bool (strict)"(error in=w103, "Value"=w102) -> ()  [unwired: 1 in, 2 out]
        n223 = property on="Running" class="Bool (strict)"(error in=w103, "Value"=w102) -> ()  [unwired: 1 in, 2 out]
      }
      event "Butt_Set": Value Change {
        w469 = T7 {"Total Time / ms"=0.0, "Image Total Collection Time"=0.0, "Image Loop time / ms"=0.0, "Peak Total Find Time"=0.0, "Peak Find Time / ms"=0.0, "Camera Rate / Hz"=0.0, "Total Number of Loops"=0.0, "Current Loop Number"=0.0, "Number of Image Loops"=0.0, "Run Mode"=0.0}  # Collection Constant
        # "Not Needed"
        # "Set up DAQ for shutters"
        # "Build image array"
        # "Set up graph display"
        # "Number of types\nTotal,\nLaser backgrounds\nIon backgrounds"
        # "Set up settings for acquire"
        n224 = event-data() -> ()  [unwired: 1 in, 6 out]
        n225 = property on="Setup?" class="Bool (strict)"(error in=w430, "Blinking"=TRUE) -> (error out=w438:errorcluster)  [unwired: 1 in, 1 out]
        n226 = property on="Session Out" class="IMAQdx (strict)"(error in=w430) -> ("Value"=w429:T3)  [unwired: 1 in, 2 out]
        n227 = property on="Run Options" class="Ring (strict)"(error in=w430) -> ("Value"=w431:u16)  [unwired: 1 in, 2 out]
        n228 = property on="Moving" class="Bool (strict)"() -> ("Value"=w445:bool)  [unwired: 2 in, 2 out]
        n229 = property on="Delay Scan?" class="Bool (strict)"(error in=w438) -> (error out=w467:errorcluster, "Value"=w468:bool)  [unwired: 1 in, 1 out]
        n230 = Unbundle By Name("DAQ Settings") -> ("Rate"=w448:dbl, "Shutter Task"=w452:refnum<k21>)
        n231 = Not(x=w445) -> (.not. x?=w443:bool)
        n232 = Not A Number/Path/Refnum?(number/path/refnum=w429) -> (NaN/Path/Refnum?=w428:bool)
        n233 = And(x=w468, y=w443) -> (x .and. y?=w444:bool)
        n234 = case shown="True" w428 {
          tunnel: [w480 w481] -> w432
          tunnel: w431 -> [w479 _]
          tunnel: w430 -> [w478 w481]
          tunnel: w429 -> [w477 _]
          frame False {
            n235 = call "VMI_clean_up_Camera.vi"("Error In"=w478, "Run Options"=w479, "Camera Session"=w477) -> ("Error Out"=w480:errorcluster)  [unwired: 4 in]
          }
          frame True {
          }
        }
        n236 = case shown="True" w444 {
          tunnel: w467 -> [w487 w493]
          tunnel: [w487 w495] -> w436
          frame False {
          }
          frame True {
            # "Set up delay control"
            n237 = control-ref of="CmdStopDelay"() -> (w489:refnum<vi>)
            n238 = property on="Delay Cluster" class="Clust (strict)"(error in=w493) -> ("Value"=w496:T11)  [unwired: 1 in, 2 out]
            n239 = call "VMI_set_Delay.vi"("Try Card"=TRUE, "Error In"=w493, "CmdStopDelay"=w489, "Delay Cluster"=w496) -> ("Error Out"=w491:errorcluster, "Delay Cluster Out"=w494:T11)  [unwired: 6 in]
            n240 = property on="Moving" class="Bool (strict)"(error in=w493, "Blinking"=TRUE) -> ()  [unwired: 1 in, 2 out]
            n241 = property on="Moving" class="Bool (strict)"(error in=w491, "Blinking"=FALSE) -> ()  [unwired: 1 in, 2 out]
            n242 = property on="Delay Cluster" class="Clust (strict)"(error in=w491, "Value"=w494) -> (error out=w495:errorcluster)  [unwired: 1 in, 1 out]
          }
        }
        n243 = Multiply(x="Acquire Time", y=w448) -> (x*y=w447:dbl)
        n244 = Bundle By Name(cluster="DAQ Settings", "Number of Samples"=w447) -> (w450:T13)
        n245 = call "VMI_Image_type_settings_array.vi"("Total Acquires"="Total Acquires", "Collection Information"="Collection Information") -> ("To Collect"=w466:i32, "Image types Bool"=w472:bool[])  [unwired: 4 in, 1 out]
        "Image types Bool" <- w472
        n246 = Unbundle By Name("Save_Files") -> ("Files to Save"=w433:bool[])
        n247 = Unbundle By Name("Camera Settings") -> ("Run Mode"=w462:u16, "X Size"=w460:dbl, "Y Size"=w459:dbl)
        n248 = call "VMI_camera_Set.vi"("error in (no error)"=w432, "Camera Settings"="Camera Settings") -> ("error out"=w442:errorcluster, "Session Out"=→"Session Out":T3, "Refnum out"=→"Image Set":T5)  [unwired: 7 in]
        n249 = Not A Number/Path/Refnum?(number/path/refnum=w452) -> (NaN/Path/Refnum?=w451:bool)
        n250 = case shown="True" w451 {
          tunnel: w450 -> [w482 w485]
          tunnel: w438 -> [w484 w486]
          tunnel: [w483 w486] -> w454
          tunnel: [w482 w485] -> w453
          frame False {
            n251 = call "DAQ_clean_daq.vi"("Error In"=w484, "DAQ Settings"=w482) -> ("Error Out"=w483:errorcluster)  [unwired: 3 in]
          }
          frame True {
          }
        }
        n252 = Boolean To (0,1)(Boolean=w472) -> (0, 1=w471:i16[])
        n253 = property on="Files to Save" class="Arr (strict)"("Value"=w433) -> ()  [unwired: 2 in, 2 out]
        n254 = Add Array Elements(numeric array=w471) -> (sum=w470:i16)
        n255 = Multiply(x="Acquire Time", y="Camera Rate / Hz") -> (x*y=w475:i32)
        n256 = Bundle By Name(cluster=w469, "Number of Image Loops"=w475, "Total Number of Loops"="Total Acquires", "Camera Rate / Hz"="Camera Rate / Hz", "Run Mode"=w462) -> (w474:T7)
        n257 = call "DAQ_set_all.vi"("Error In"=w454, "DAQ Settings"=w453) -> ("Error Out"=w455:errorcluster, "DAQ Out"=w456:T13)  [unwired: 2 in]
        n258 = property on="DAQ Settings" class="Clust (strict)"(error in=w455, "Value"=w456) -> (error out=w440:errorcluster)  [unwired: 1 in, 1 out]
        n259 = Merge Errors(w442, w440, w436) -> (w441:errorcluster)
        n260 = property on="Collection Results" class="Clust (strict)"("Value"=w474) -> ()  [unwired: 2 in, 2 out]
        n261 = property on="Counts per image" class="XYGraph (strict)"("LegNumRows"=w470) -> ()  [unwired: 2 in, 2 out]
        n262 = case shown="No Error" w441 {
          tunnel: w441 -> [w504 w510]
          tunnel: [w501 w508] -> w439
          frame No Error {
            # "Mark setup"
            # "Sets up queues\nto allow acquisition at same time as analysis"
            # "Set up queues"
            n263 = call "VMI_queue_set_up_arrays.vi"("error in (no error)"=w504, "Number of Queues"=3) -> ("error out"=w503:errorcluster, "Stop"=→"Queue Check":bool, "Queue Array"=→"Queue Array":T4[])  [unwired: 1 in]
            n264 = property on="Setup?" class="Bool (strict)"(error in=w503, "Value"=TRUE ("Setup?"), "Blinking"=FALSE) -> (error out=w501:errorcluster)  [unwired: 1 in, 1 out]
            n265 = property on="Collect" class="Bool (strict)"(error in=w501, "DisabledEnum"=T18."Enabled" ("Disabled")) -> (error out=w499:errorcluster)  [unwired: 1 in, 1 out]
            n266 = property on="Butt_Set" class="Bool (strict)"(error in=w499, "Value"=FALSE ("Butt_Set")) -> ()  [unwired: 1 in, 2 out]
          }
          frame Error {
            # "Camera set up error"
            n267 = call <vilib>:"General Error Handler.vi"("error in (no error)"=w510) -> ("error out"=w509:errorcluster)  [unwired: 10 in, 4 out]
            n268 = call <vilib>:"Clear Errors.vi"("error in (no error)"=w509) -> ("error out"=w508:errorcluster)  [unwired: 5 in, 1 out]
          }
        }
        n269 = call "VMI_create_arrays.vi"("Collection Information"="Collection Information", "Ysize"=w459, "Xsize"=w460) -> ("Big_image Array"=→"Big_image Array":i16[][][], "Image Array"=w461:dbl[][])  [unwired: 7 in]
        n270 = for {
          N: w466 -> [_]
          tunnel: "Collection Information" -> [w513] mode=indexing
          i -> [w514]
          n271 = Unbundle By Name(w513) -> ("Collect"=w511:bool, "Type"=w512:string)
          n272 = property on="Counts per image" class="XYGraph (strict)"("Active Plot"=w514, "Plot.Visible?"=w511, "Plot.Plot Name"=w512) -> ()  [unwired: 2 in, 2 out]
        }
        n273 = property on="SIgnal Image Array" class="Arr (strict)"("Value"=w461) -> ()  [unwired: 2 in, 2 out]
        n274 = property on="Bakc Image" class="Arr (strict)"("Value"=w461) -> ()  [unwired: 2 in, 2 out]
        n275 = property on="Bakc Image2" class="Arr (strict)"("Value"=w461) -> ()  [unwired: 2 in, 2 out]
      }
      event "Save All": Value Change {
        n276 = event-data() -> ("CtlRef"=w517:refnum<vi>, "NewVal"=w515:bool)  [unwired: 1 in, 4 out]
        n277 = case shown="True" w515 {
          tunnel: w518 -> [w520 w541]
          tunnel: w517 -> [_ w539]
          tunnel: [w520 w528] -> w516
          frame False {
          }
          frame True {
            # "If changed to True set up next file name"
            n278 = property on="Backup Path" class="Path"() -> ("Value"=w526:path)  [unwired: 2 in, 2 out]
            n279 = property on="Main Directory" class="Path"() -> ("Value"=w537:path)  [unwired: 2 in, 2 out]
            n280 = property on="Savechoose" class="Bool (strict)"() -> ("Value"=w536:bool)  [unwired: 2 in, 2 out]
            n281 = call "VMI_set_date_path.vi"("Value"=w537, "Remote path 2"=w526, "error in (no error)"=w541) -> ("appended path"=w535:path, "New Date Name"=w529:string, "appended path 2"=w524:path, "error out"=w522:errorcluster)
            n282 = case shown="True" w536 {
              tunnel: w535 -> [w563 _]
              tunnel: [w563 w564] -> w532
              frame False {
              }
              frame True {
                n283 = call "File Dialog"() -> ("selected path"=w564:path)  [unwired: 12 in, 3 out]
              }
            }
            n284 = property on="Current File Date and endings" class="Str"("Value"=w529) -> ()  [unwired: 2 in, 2 out]
            n285 = control-ref of="Save All"() -> (w540:refnum<vi>)
            n286 = Equal?(x=w540, y=w539) -> (x = y?=w538:bool)
            n287 = property on="Save Path" class="Path"("Value"=w532) -> ()  [unwired: 2 in, 2 out]
            n288 = property on="Collection Information" class="Arr (strict)"() -> ("Value"=w530:T10[])  [unwired: 2 in, 2 out]
            n289 = property on="Remote" class="Bool (strict)"() -> ("Value"=w525:bool)  [unwired: 2 in, 2 out]
            n290 = case shown="True" w538 {
              tunnel: w522 -> [w565 w578]
              tunnel: [w565 w576] -> w521
              tunnel: w532 -> [_ w577]
              tunnel: w529 -> [_ w574]
              tunnel: w530 -> [_ w571]
              tunnel: w524 -> [_ w567]
              tunnel: w525 -> [_ w566]
              frame False {
              }
              frame True {
                n291 = property on="Image Info Acqu" class="Clust (strict)"() -> ("Value"=w569:T8)  [unwired: 2 in, 2 out]
                n292 = property on="Histogram_array" class="Arr (strict)"() -> ("Value"=w575:i32[][])  [unwired: 2 in, 2 out]
                n293 = property on="Hist_full" class="Arr (strict)"() -> ("Value"=w572:dbl[][][])  [unwired: 2 in, 2 out]
                n294 = property on="Peaks" class="Arr (strict)"() -> ("Value"=w573:T1[])  [unwired: 2 in, 2 out]
                n295 = call "VMI_save_Files_backup.vi"("appended path"=w577, "ChangeFile"=TRUE, "Hist_full"=w572, "Image Info"=w569, "Histogram_array"=w575, "Current File Date"=w574, "Remote Save?"=w566, "Collection Information"=w571, "Save"="Files to Save", "error in (no error)"=w578, "Remote_path"=w567, "Peaks"=w573) -> ("error out"=w576:errorcluster)  [unwired: 3 in]
              }
            }
            n296 = case shown="True" "Log File" {
              tunnel: w521 -> [w554 w562]
              tunnel: w532 -> [_ w561]
              tunnel: w530 -> [_ w558]
              tunnel: w525 -> [_ w557]
              tunnel: w524 -> [_ w556]
              tunnel: [w554 w555] -> w523
              frame False {
              }
              frame True {
                n297 = property on="Scan Set up" class="Clust (strict)"() -> ("Value"=w560:T9)  [unwired: 2 in, 2 out]
                n298 = property on="Delay Cluster" class="Clust (strict)"() -> ("Value"=w559:T11)  [unwired: 2 in, 2 out]
                n299 = call "Scan_ctrl.vi"("Scan Set up"=w560, "Remote?"=w557, "appended path"=w561, "Value"=w558, "Delay Cluster"=w559, "error in (no error)"=w562, "Remotepath"=w556) -> ("error out"=w555:errorcluster)  [unwired: 1 out]
              }
            }
            n300 = case shown="True" "Database" {
              tunnel: w521 -> [w542 w545]
              tunnel: w530 -> [_ w549]
              tunnel: w529 -> [_ w548]
              tunnel: [w542 w544] -> w527
              frame False {
              }
              frame True {
                n301 = property on="Scan Type" class="Ring (strict)"(error in=w545) -> ("RingText.Text"=w547:string)  [unwired: 1 in, 2 out]
                n302 = property on="Chemical" class="Str"() -> ("Value"=w546:string)  [unwired: 2 in, 2 out]
                n303 = call "Build_database_info.vi"("Collection Info Array"=w549, "Chemical"=w546, "RingText.Text"=w547, "New Date Name"=w548) -> ("Data to add"=w543:T24)  [unwired: 7 in]
                n304 = disable-structure shown="Disabled" {
                  disable-tunnel: w545 -> [w552 w553]
                  disable-tunnel: [w551 w553] -> w544
                  disable-tunnel: w543 -> [w550 _]
                  frame Disabled {
                    n305 = call "Save_local_database.vi"("error in (no error)"=w552, "Data to add"=w550) -> ("error out"=w551:errorcluster)  [unwired: 3 in]
                  }
                  frame Enabled {
                  }
                }
              }
            }
            n306 = Merge Errors(w521, w527, w523) -> (w528:errorcluster)
            n307 = property on="Save All" class="Bool (strict)"(error in=w521, "Value"=FALSE ("Save All")) -> ()  [unwired: 1 in, 2 out]
          }
        }
        n308 = property on="Image Info Acqu" class="Clust (strict)" props=["Value"]() -> ()  [unwired: 2 in, 3 out]
      }
      event Value Change {
        w579 = T1 {"Peaks"=[], "size"=0, "Title"=""}  # Peak Controls
        w582 = T10 {"Type"="", "LaserWave1"=0.0, "Shutter1"=FALSE, "LaserWave2"=0.0, "Shutter2"=FALSE, "FileEnd"="", "Collect"=FALSE}  # Collection Settings
        # "Set up collection information"
        n309 = event-data() -> ("NewVal"=w583:u16)  [unwired: 1 in, 5 out]
        n310 = case shown="2" w583 {
          selector: w583 -> [_ _ w643 w668]
          tunnel: w582 -> [w600 w619 w650 w677]
          tunnel: w581 -> [w591 w614 w636 w672]
          tunnel: [w590 w611 w641 w666] -> w580
          tunnel: w579 -> [w589 w609 w638 w659]
          frame 0, Default {
            (unwired) 0.0 ("LaserWave2")
            (unwired) 0.0 ("LaserWave1")
            # "This is a normal collection so only one file"
            n311 = Bundle By Name(cluster=w600, "Type"="Signal and Background", "Shutter1"=TRUE ("Chopped1"), "Shutter2"=FALSE ("Chopped2"), "FileEnd"="_SignalBack", "Collect"=TRUE) -> (w594:T10)
            n312 = Bundle By Name(cluster=w589, "Title"="Signal Background") -> (w587:T1)
            n313 = Build Array(w594) -> (w593:T10[])
            n314 = Build Array(w587) -> (w586:T1[])
            n315 = property on="Collection Information" class="Arr (strict)"(error in=w591, "Value"=w593) -> (error out=w585:errorcluster)  [unwired: 1 in, 1 out]
            n316 = property on="Peaks" class="Arr (strict)"(error in=w585, "Value"=w586) -> (error out=w584:errorcluster)  [unwired: 1 in, 1 out]
            n317 = property on="Delay Scan?" class="Bool (strict)"(error in=w584, "Value"=FALSE ("Delay Scan")) -> (error out=w590:errorcluster)  [unwired: 1 in, 1 out]
          }
          frame 1 {
            w612 = FALSE ("Delay Scan")
            (unwired) 0.0 ("LaserWave1")
            (unwired) 0.0 ("LaserWave1")
            (unwired) 0.0 ("LaserWave2")
            (unwired) 0.0 ("LaserWave1")
            # "Second file - one colour blocked"
            # "2 colour normal collection - so two background files"
            n318 = Bundle By Name(cluster=w619, "Type"="Signal and Background", "Shutter1"=TRUE ("Chopped1"), "Shutter2"=TRUE ("Chopped2"), "FileEnd"="_SignalBack", "Collect"=TRUE) -> (w618:T10)
            n319 = Bundle By Name(cluster=w619, "Type"="Background1", "Shutter1"=TRUE ("Chopped1"), "Shutter2"=FALSE ("Chopped2"), "FileEnd"="_LasBack1", "Collect"=TRUE) -> (w617:T10)
            n320 = Bundle By Name(cluster=w619, "Type"="Background2", "Shutter1"=FALSE ("Chopped1"), "Shutter2"=TRUE ("Chopped2"), "FileEnd"="_LasBack2", "Collect"=TRUE) -> (w616:T10)
            n321 = Bundle By Name(cluster=w609, "Title"="Signal Background") -> (w608:T1)
            n322 = Bundle By Name(cluster=w609, "Title"="Background1") -> (w607:T1)
            n323 = Bundle By Name(cluster=w609, "Title"="Background2") -> (w606:T1)
            n324 = Build Array(w618, w617, w616) -> (w615:T10[])
            n325 = property on="Collection Information" class="Arr (strict)"(error in=w614, "Value"=w615) -> (error out=w602:errorcluster)  [unwired: 1 in, 1 out]
            n326 = Build Array(w608, w607, w606) -> (w603:T1[])
            n327 = property on="Peaks" class="Arr (strict)"(error in=w602, "Value"=w603) -> (error out=w601:errorcluster)  [unwired: 1 in, 1 out]
            n328 = property on="Delay Scan?" class="Bool (strict)"(error in=w601, "Value"=w612) -> (error out=w613:errorcluster)  [unwired: 1 in, 1 out]
            n329 = property on="Accurate Scan" class="Bool (strict)"(error in=w613, "Value"=w612) -> (error out=w611:errorcluster)  [unwired: 1 in, 1 out]
          }
          frame 2 {
            (unwired) 0.0 ("LaserWave2")
            (unwired) 0.0 ("LaserWave1")
            # "This is a delay scan with two colours - only collect counts"
            n330 = Bundle By Name(cluster=w638, "Title"="Signal Background") -> (w639:T1)
            n331 = Bundle By Name(cluster=w650, "Type"="Signal and Background", "Shutter1"=TRUE ("Chopped1"), "Shutter2"=TRUE ("Chopped2"), "FileEnd"="_SignalBack", "Collect"=TRUE) -> (w649:T10)
            n332 = Build Array(w639) -> (w637:T1[])
            n333 = property on="Peaks" class="Arr (strict)"(error in=w636, "Value"=w637) -> (error out=w635:errorcluster)  [unwired: 1 in, 1 out]
            n334 = Build Array(w649) -> (w648:T10[])
            n335 = property on="Collection Information" class="Arr (strict)"(error in=w635, "Value"=w648) -> (error out=w647:errorcluster)  [unwired: 1 in, 1 out]
            n336 = property on="Delay Scan?" class="Bool (strict)"(error in=w647, "Value"=TRUE ("Delay Scan")) -> (error out=w645:errorcluster)  [unwired: 1 in, 1 out]
            n337 = Equal?(x=w643, y=u16 3) -> (x = y?=w644:bool)
            n338 = property on="Accurate Scan" class="Bool (strict)"(error in=w645, "Value"=w644) -> (error out=w641:errorcluster)  [unwired: 1 in, 1 out]
          }
          frame 3 {
            (unwired) 0.0 ("LaserWave1")
            (unwired) 0.0 ("LaserWave1")
            (unwired) 0.0 ("LaserWave2")
            (unwired) 0.0 ("LaserWave1")
            # "Second file - one colour blocked"
            # "This is a delay scan with two colours - accurate move and collect repeatedly"
            n339 = Bundle By Name(cluster=w677, "Type"="Signal and Background", "Shutter1"=TRUE ("Chopped1"), "Shutter2"=TRUE ("Chopped2"), "FileEnd"="_SignalBack", "Collect"=TRUE) -> (w676:T10)
            n340 = Bundle By Name(cluster=w677, "Type"="Background1", "Shutter1"=TRUE ("Chopped1"), "Shutter2"=FALSE ("Chopped2"), "FileEnd"="_LasBack1", "Collect"=TRUE) -> (w675:T10)
            n341 = Bundle By Name(cluster=w659, "Title"="Signal Background") -> (w664:T1)
            n342 = Bundle By Name(cluster=w677, "Type"="Background2", "Shutter1"=FALSE ("Chopped1"), "Shutter2"=TRUE ("Chopped2"), "FileEnd"="_LasBack2", "Collect"=TRUE) -> (w674:T10)
            n343 = Bundle By Name(cluster=w659, "Title"="Background1") -> (w663:T1)
            n344 = Bundle By Name(cluster=w659, "Title"="Background2") -> (w662:T1)
            n345 = Build Array(w676, w675, w674) -> (w673:T10[])
            n346 = Build Array(w664, w663, w662) -> (w658:T1[])
            n347 = property on="Collection Information" class="Arr (strict)"(error in=w672, "Value"=w673) -> (error out=w657:errorcluster)  [unwired: 1 in, 1 out]
            n348 = property on="Peaks" class="Arr (strict)"(error in=w657, "Value"=w658) -> (error out=w656:errorcluster)  [unwired: 1 in, 1 out]
            n349 = property on="Delay Scan?" class="Bool (strict)"(error in=w656, "Value"=TRUE ("Delay Scan")) -> (error out=w670:errorcluster)  [unwired: 1 in, 1 out]
            n350 = Equal?(x=w668, y=u16 3) -> (x = y?=w669:bool)
            n351 = property on="Accurate Scan" class="Bool (strict)"(error in=w670, "Value"=w669) -> (error out=w666:errorcluster)  [unwired: 1 in, 1 out]
          }
        }
      }
      event "Butt_Load": Value Change {
        # "Load the point file"
        n352 = event-data() -> ()  [unwired: 1 in, 6 out]
        n353 = property on="Loaded" class="Bool (strict)"(error in=w697, "Value"=FALSE ("Loaded")) -> ()  [unwired: 1 in, 2 out]
        n354 = call "File Dialog2"("start path"="Analysis Path", "error in"=w697) -> ("selected path"=w694:path, "cancelled"=w693:bool, "error out"=w696:errorcluster)  [unwired: 10 in, 1 out]
        n355 = case shown="False" w693 {
          tunnel: [w704 w718] -> w699
          tunnel: w696 -> [w702 w718]
          tunnel: w694 -> [w701 _]
          frame False {
            # "Load file"
            n356 = property on="Analysis Path" class="Path"("Value"=w701) -> ()  [unwired: 2 in, 2 out]
            n357 = Read from Text File(file (use dialog)=w701, error in=w702) -> (text=w705:string, error out=w703:errorcluster)  [unwired: 2 in, 2 out]
            n358 = case shown="No Error" w703 {
              tunnel: w705 -> [w716 _]
              tunnel: w703 -> [w709 w717]
              tunnel: [w708 w717] -> w704
              frame No Error {
                # "Convert to point array"
                n359 = call "Point_string_to_points.vi"("Points String"=w716) -> ("Points"=w714:cluster{"X":sgl, "Y":sgl}[], "Num Points"=→"Num Points":i32)  [unwired: 3 in]
                "Loaded Points" <- w714
                n360 = Unbundle By Name("Image Info") -> ("X size"=w710:dbl, "Y size"=w711:dbl)
                n361 = call "VMI_create_image_from_points.vi"("New Array"=TRUE, "Image Info"="Image Info", "Points"=w714) -> ("Image Array"=w707:i16[][])  [unwired: 2 in]
                "Image Array" <- w707
                n362 = property on="Loaded" class="Bool (strict)"("Value"=TRUE ("Loaded")) -> ()  [unwired: 2 in, 2 out]
                n363 = property on="Intensity Graph" class="IntGraph (strict)"(error in=w709, "XScale.Maximum"=w710, "YScale.Maximum"=w711) -> (error out=w708:errorcluster)  [unwired: 1 in, 1 out]
                n364 = property on="Intensity Graph" class="IntGraph (strict)"("Value"=w707) -> ()  [unwired: 2 in, 2 out]
              }
              frame Error {
              }
            }
          }
          frame True {
          }
        }
      }
      event Value Change {
        w720 = FALSE ("Value")
        n365 = event-data() -> ("NewVal"=w724:bool)  [unwired: 1 in, 5 out]
        n366 = case shown="True" w724 {
          tunnel: w723 -> [w725 w730]
          tunnel: [w725 w727] -> w721
          frame False {
          }
          frame True {
            w732 = TRUE ("SetV?")
            w728 = FALSE ("Blinking")
            w731 = TRUE ("Blinking")
            # "Check position"
            n367 = property on="Delay Cluster" class="Clust (strict)"(error in=w730) -> ("Value"=w735:T11)  [unwired: 1 in, 2 out]
            n368 = property on="Moving" class="Bool (strict)"(error in=w730, "Blinking"=w731) -> ()  [unwired: 1 in, 2 out]
            n369 = property on="Delay Moving" class="Bool (strict)"(error in=w730, "Blinking"=w731) -> ()  [unwired: 1 in, 2 out]
            n370 = control-ref of="CmdStopDelay"() -> (w733:refnum<vi>)
            n371 = control-ref of="Postion / mm"() -> (w734:refnum<vi>)
            n372 = call "VMI_move_wait_PI.vi"("SetV?"=w732, "Move and Wait?"=w732, "Delay Cluster"=w735, "Error In"=w730, "Stop ref"=w733, "Postion / mm"=w734) -> ("error out"=w729:errorcluster)  [unwired: 5 in]
            n373 = call <vilib>:"Clear Errors.vi"("error in (no error)"=w729, "specific error code to clear (0: all)"=10) -> ("error out"=w727:errorcluster)  [unwired: 4 in, 1 out]
            n374 = property on="Moving" class="Bool (strict)"(error in=w727, "Blinking"=w728) -> ()  [unwired: 1 in, 2 out]
            n375 = property on="Delay Moving" class="Bool (strict)"(error in=w727, "Blinking"=w728) -> ()  [unwired: 1 in, 2 out]
          }
        }
        n376 = property on="CmdMovDelay" class="Bool (strict)"(error in=w721, "Value"=w720) -> (error out=w719:errorcluster)  [unwired: 1 in, 1 out]
        n377 = property on="CmdStopDelay" class="Bool (strict)"(error in=w719, "Value"=w720) -> ()  [unwired: 1 in, 2 out]
      }
      event "Stop All", "Stop All Anly": Value Change {
        w744 = FALSE ("Setup?")
        n378 = event-data() -> ()  [unwired: 1 in, 6 out]
        n379 = property on="Setup?" class="Bool (strict)"() -> ("Value"=w746:bool)  [unwired: 2 in, 2 out]
        n380 = case shown="True" w746 {
          tunnel: w747 -> [w749 w751]
          tunnel: [w749 w750] -> w740
          frame False {
          }
          frame True {
            # "If setup clean queue"
            n381 = property on="Queue Array" class="Arr (strict)"() -> ("Value"=w752:T4[])  [unwired: 2 in, 2 out]
            n382 = call "VMI_queue_clean_up_arrays.vi"("error in (no error)"=w751, "Queue Array"=w752) -> ("error out"=w750:errorcluster)  [unwired: 1 in]
          }
        }
        n383 = property on="Image Set" class="IMAQImage (strict)"() -> ("Value"=w745:T5)  [unwired: 2 in, 2 out]
        n384 = call "Close connection if open.vi"("System no."=1, "error in"=w740) -> ("error out"=w737:errorcluster)  [unwired: 1 in, 16 out]
        n385 = property on="DAQ Settings" class="Clust (strict)"(error in=w740) -> ("Value"=w743:T13)  [unwired: 1 in, 2 out]
        n386 = call "IMAQ Dispose"("Image"=w745, "error in (no error)"=w740) -> ()  [unwired: 4 in, 1 out]
        n387 = property on="Setup?" class="Bool (strict)"(error in=w740, "Value"=w744) -> (error out=w742:errorcluster)  [unwired: 1 in, 1 out]
        n388 = property on="Collect" class="Bool (strict)"(error in=w742, "Value"=w744) -> ()  [unwired: 1 in, 2 out]
        n389 = property on="Moving" class="Bool (strict)"(error in=w737, "Value"=FALSE) -> ()  [unwired: 1 in, 2 out]
        n390 = call "DAQ_clean_daq.vi"("Error In"=w742, "DAQ Settings"=w743) -> ("Error Out"=w741:errorcluster)  [unwired: 3 in]
        n391 = Merge Errors(w741, w737) -> (w738:errorcluster)
      }
      event "Save anl": Value Change {
        # "Save the image file out"
        n392 = event-data() -> ()  [unwired: 1 in, 6 out]
        n393 = property on="Analysis Path" class="Path"(error in=w757) -> (error out=w754:errorcluster, "Value"=w758:path)  [unwired: 1 in, 1 out]
        n394 = call "VMI_save_IF32_path.vi"("Analysis Path"=w758) -> ("cancelled"=w755:bool, "selected path"=w756:path)  [unwired: 1 in]
        n395 = case shown="False" w755 {
          tunnel: w756 -> [w763 _]
          tunnel: w754 -> [w765 w773]
          tunnel: [w760 w773] -> w753
          frame False {
            n396 = property on="Image Info" class="Clust (strict)"() -> ("Value"=w769:T8)  [unwired: 2 in, 2 out]
            n397 = Strip Path(path=w763) -> (name=w771:string)  [unwired: 1 out]
            n398 = property on="Image Array" class="Arr (strict)"(error in=w765) -> (error out=w761:errorcluster, "Value"=w764:i16[][])  [unwired: 1 in, 1 out]
            n399 = Transpose 2D Array(2D array=w764) -> (transposed array=w759:i16[][])
            n400 = Bundle By Name(cluster=T22 {"File Name"="080916aa", "Time"="Hammer", "Date"="Now", "Size"=""} ("Cluster"), "File Name"=w771, "Time"="00:00:00", "Date"="?", "Size"="16") -> (w770:T22)
            n401 = call "VMI_save_IF32_format.vi"("Image Array"=w759, "Image Info"=w769, "Header Cluster"=w770) -> ("File String"=w762:string)  [unwired: 2 in]
            n402 = Write to Text File(file (use dialog)=w763, text=w762, error in=w761) -> (error out=w760:errorcluster)  [unwired: 1 in, 2 out]
          }
          frame True {
          }
        }
      }
    }
  }
  n403 = call <vilib>:"Simple Error Handler.vi"("error in (no error)"=w38) -> ("error out"=→"Error Out":errorcluster)  [unwired: 4 in, 4 out]
  "Setup?" <- "Butt_Set"
